vi "Process.vi"(8 "error in":errorcluster, 11 "Inst UI.Attocube-3DR":refnum<class "Inst UI.Attocube-3DR.lvclass">) -> (0 "error out":errorcluster, 3 "Inst UI.Attocube-3DR out":refnum<class "Inst UI.Attocube-3DR.lvclass">)   [LabVIEW 2019, in "Inst UI.Attocube-3DR.lvclass"]
doc: "---------------------------------------------------------------\nJKI State Machine Objects™\nhttp://jki.net/state-machine-objects/\nCopyright (C) 2005-2015, JKI <info@jki.net>\nALL RIGHTS RESERVEDJKI State Machine Objects (SMO) 1.0.0.5\nJKI - JKI\nCopyright (c) 2016, JKI"
uses:
  Inst UI.Attocube-3DR.lvclass
  C:/Program Files (x86)/National Instruments/LabVIEW 2019/vi.lib/JKI/JKI SMO/SMO/SMO.lvclass
  C:/Program Files (x86)/National Instruments/LabVIEW 2019/user.lib/LevyLab/Instrument Framework/SMOs/Instrument UI/Instrument UI.lvclass
  C:/Program Files (x86)/National Instruments/LabVIEW 2019/vi.lib/JKI/JKI SMO/SMO.UI/SMO.UI.lvclass
  Inst.Attocube-3DR/Typedefs/Inst.Attocube-3DR.Inputs--Cluster.ctl
  Inst.Attocube-3DR/Typedefs/Inst.Attocube-3DR.getAll--Cluster.ctl
  Inst.Attocube-3DR/Inst.Attocube-3DR.lvclass
  C:/Program Files (x86)/National Instruments/LabVIEW 2019/user.lib/LevyLab/Instrument Framework/SMOs/Instrument/Instrument.lvclass
  Inst UI.Attocube-3DR.UI--Cluster.ctl
  Inst.Attocube-3DR/Typedefs/Inst.Attocube-3DR.Configuration--Cluster.ctl
  <userlib>/LevyLab/Instrument Framework/SMOs/Configuration/Configuration.lvclass
  <userlib>/LevyLab/Instrument Framework/SMOs/RemoteControl/Typedefs/Message--Cluster.ctl
  <userlib>/LevyLab/Instrument Framework/SMOs/Instrument UI/Instrument UI.lvclass/Instrument UI.ctl
  Inst.Attocube-3DR/Inst.Attocube-3DR.lvclass/Inst.Attocube-3DR.ctl
  <vilib>/JKI/JKI SMO/SMO/SMO.lvclass/SMO.ctl
  <userlib>/LevyLab/Instrument Framework/SMOs/Configuration/Configuration.lvclass/Configuration.ctl
  <userlib>/LevyLab/Instrument Framework/SMOs/Instrument/Instrument.lvclass/Instrument.ctl
  <userlib>/LevyLab/Instrument Framework/SMOs/Instrument/Typedefs/Client Type--Enum.ctl
  862ff513-51e6-4ac6-ad45-748a4df68803.vi
  048e63fc-1edb-448e-8f4f-f5318f48fab1.vi
  6f37eb51-0e53-4202-aa6b-7eeea6d1e979.vi
  436f7c45-6ac9-4282-a393-d7a55f5a58f8.vi
  53aa8742-20c4-45a9-88cf-31145ab324ca.vi
  a7dc0b2d-59f7-45fe-b3a9-fa8b57d3da12.vi
  4acd7b6f-92e7-4c4b-af86-ffc31bbcab9e.vi
  e11c7c74-b7c8-4525-a80a-41ba14629eb8.vi
  b80c2030-d11d-4dfa-959a-d9fba43c27d5.vi
  9f19d11c-c97f-4e63-8b6c-fa81cfd939c9.vi
  a687013f-834b-44a6-a6f3-22fcdf7d7604.vi
  d852ea7b-884f-4206-b538-26d982e90c02.vi
  6e0f0dad-eeb2-4aa9-8821-537bff27e402.vi
  351b4355-bf82-4134-82c7-732762f03f32.vi
  2787704c-df89-403c-943f-ae81abeff9f3.vi
  16be1e38-bb79-47d8-99ba-5a82125cb6c1.vi
  c0fbbb13-e8ef-413d-99ab-b1af3e8c1fc5.vi
  7278661c-b813-447f-a135-8e1ce543f15b.vi
  77de4e95-45da-414c-9291-629979477714.vi
  fc3948ed-5b37-4c89-8f64-66d1f3e9a865.vi
  89faabad-b894-427a-af3b-2e65de9d785f.vi
  6d94cbbf-a9ac-4f89-8b31-e4a871a3db8e.vi
  914930c5-8721-4ac6-bb66-38959b5d5002.vi
  a5ebc035-e685-45b2-a8ec-287c660a7532.vi
  c3992a28-0ace-4d19-8331-9b0e91a8ecb4.vi
  9e101b16-2f91-4f38-b95c-e3ff51136ff6.vi
  99d154c9-cb9c-4973-bc75-571f88aa4a64.vi
  1056dc58-91e4-4912-a0c3-223d5a7ab089.vi
  1b9e2014-56cb-49fc-a14d-f0a40d2771d4.vi
  151c6d9c-9f8f-4aeb-92d7-c211fa7e2556.vi
  b6919943-735e-4033-8b93-0939513f520d.vi
  d99a13ac-48ea-4f37-a989-76a16f5559e3.vi
  f1f28e6d-5397-42c6-984c-224e3dbbef4b.vi
  f68b141c-1cbc-4bee-b372-ea377a2360ca.vi
  32104498-4a8d-4312-9ef2-1fa6833386a6.vi
  f6d8fc86-ed5e-4e4c-a4d2-98ad122425f6.vi
  09e9697b-516c-49fb-b2dc-692589121b6f.vi
  <vilib>/JKI/JKI SMO/SMO/Private/ReftoDVR--SMO.vi
  09e9697b-516c-49fb-b2dc-692589121b6f.vi/3ffc5513-9bd7-4c71-8aef-4de823704d0f.vi
  09e9697b-516c-49fb-b2dc-692589121b6f.vi/3ffc5513-9bd7-4c71-8aef-4de823704d0f.vi/f6b0c238-dc1e-49e3-8a4e-b8369e72da79.vi
  <userlib>/LevyLab/Instrument Framework/SMOs/Instrument/API/Send and Receive.vi
  09e9697b-516c-49fb-b2dc-692589121b6f.vi/3ffc5513-9bd7-4c71-8aef-4de823704d0f.vi/a86054fe-ddd2-4fec-9414-8fc011e039af.vi
  <userlib>/LevyLab/Instrument Framework/SMOs/Instrument/Private/Get Client Type.vi
  09e9697b-516c-49fb-b2dc-692589121b6f.vi/3ffc5513-9bd7-4c71-8aef-4de823704d0f.vi/f6b0c238-dc1e-49e3-8a4e-b8369e72da79.vi/2c6d981d-8b19-4ad3-942a-196c15fa35a5.vi
  09e9697b-516c-49fb-b2dc-692589121b6f.vi/3ffc5513-9bd7-4c71-8aef-4de823704d0f.vi/f6b0c238-dc1e-49e3-8a4e-b8369e72da79.vi/45ea1e73-aa8f-40ed-94ca-4b399240c4c1.vi
  09e9697b-516c-49fb-b2dc-692589121b6f.vi/3ffc5513-9bd7-4c71-8aef-4de823704d0f.vi/a86054fe-ddd2-4fec-9414-8fc011e039af.vi/b596e68e-c0c0-4011-92a4-140a9372dc21.vi
  09e9697b-516c-49fb-b2dc-692589121b6f.vi/3ffc5513-9bd7-4c71-8aef-4de823704d0f.vi/a86054fe-ddd2-4fec-9414-8fc011e039af.vi/f487987f-ebb9-4243-a7de-9c5ef0d70179.vi
  09e9697b-516c-49fb-b2dc-692589121b6f.vi/3ffc5513-9bd7-4c71-8aef-4de823704d0f.vi/a86054fe-ddd2-4fec-9414-8fc011e039af.vi/b596e68e-c0c0-4011-92a4-140a9372dc21.vi/c9a861e6-b5dc-4bd8-be54-56d7304e8390.vi
  09e9697b-516c-49fb-b2dc-692589121b6f.vi/3ffc5513-9bd7-4c71-8aef-4de823704d0f.vi/a86054fe-ddd2-4fec-9414-8fc011e039af.vi/b596e68e-c0c0-4011-92a4-140a9372dc21.vi/402cfb81-c0e6-461e-a8cb-63e9dc5cb757.vi
  <vilib>/JDP Science/JSONtext/Variant to JSON Text.vi
  <userlib>/LevyLab/Instrument Framework/SMOs/Instrument/Private/Get RC Connection Status.vi
  <userlib>/LevyLab/Instrument Framework/SMOs/Instrument/API/Enum to String.vi
  <userlib>/LevyLab/Instrument Framework/SMOs/RemoteControl/API/Send and Receive.vi
  <vilib>/Utility/Data Type/Get Type Information.vi
  <vilib>/JDP Science/JSONtext/JSON text to Variant.vi
  <vilib>/National Instruments/GUID Generator/Guid Generator.vi
  <userlib>/LevyLab/Instrument Framework/SMOs/Instrument/Private/Instrument.MessageFromProcess.EventStructure.vi
  <vilib>/JDP Science/JSONtext/LVClass Serializer/JSONtext LVClass Serializer.lvclass
  <userlib>/LevyLab/Instrument Framework/SMOs/Instrument/Instrument.lvclass
  <userlib>/LevyLab/Instrument Framework/SMOs/Instrument UI/Instrument UI.lvclass
  <vilib>/JKI/JKI SMO/SMO/SMO.lvclass
  <vilib>/JKI/JKI SMO/SMO.UI/SMO.UI.lvclass
  <userlib>/LevyLab/Instrument Framework/SMOs/RemoteControl/RemoteControl.lvclass
  69065371-e868-4e0f-beed-6b6e2b461ff4.vi
  C:/Program Files (x86)/National Instruments/LabVIEW 2019/user.lib/LevyLab/Instrument Framework/Instrument Types/VSource/Instrument.VSource.lvclass
panel:
  in  "Exit":bool
  out "Axis 1: Current Position (°)":i32
  out "Axis 1: rot. count":i32
  out "Axis 1: Capacitance [nF]":i32
  out "Axis 2: Capacitance [nF]":i32
  out "Axis 1: speed (°/s)":i32
  out "Axis 1: StepWidth":i32
  out "Axis 2: StepWidth":i32
  out "Axis 2: speed (°/s)":i32
  out "Axis 2: rot. count":i32
  out "last move time":timestamp
  out "axis 1:\nCurrent position [µm/°/m°] 2":i32(knob) scale=65.0..270.0
  in  "set static amplitude\nwhen moving":bool
  in  "static amplitude (mV)":dbl=2.0 min=0.001 max=2.0 format="%#_13g"
  in  "axis 2:\nStop moving":bool
  in  "axis 1:\nStop moving":bool
  in  "axis 2:\nstop detection":bool
  in  "axis 1:\nstop detection":bool
  in  "axis 2:\nOutput":bool
  in  "axis 1:\ncontrol mode":enum16{"speed", "amplitude", "step size"}(ring)=enum."amplitude"
  in  "axis 2:\ncontrol mode":enum16{"speed", "amplitude", "step size"}(ring)=enum."amplitude"
  in  "axis 1:\nOutput":bool
  in  "axis 2:\ncap. measure":bool
  in  "axis 1:\ncap. measure":bool
  out "axis 2:\nCurrent position [µm/°/m°] 2":i32(knob) scale=5.0..320.0
  in  "axis 2:\nFrequency [Hz]":i32=800 min=0 max=20000 format="%.0fHz"
  in  "axis 1:\nFrequency [Hz]":i32=800 min=0 max=20000 format="%.0fHz"
  in  "axis 2:\nDCLevel [V]":dbl min=0.0 max=140.0 step=0.001 format="%.3f"
  in  "axis 1:\nDCLevel [V]":dbl min=0.0 max=140.0 step=0.001 format="%.3f"
  in  "axis 2:\nAmplitude [V]":dbl=35.0 min=0.0 max=150.0 format="%.3gV"
  in  "axis 1:\nAmplitude [V]":dbl=40.0 min=0.0 max=150.0 format="%.3gV"
  in  "axis 2:\ncontinuous back":bool
  in  "axis 2:\ncontinuous fwd":bool
  in  "axis 1:\ncontinuous back":bool
  in  "axis 1:\ncontinuous fwd":bool
  in  "axis 2:\nsingle step fwd":bool
  in  "axis 2:\nsingle step back":bool
  in  "axis 1:\nsingle step back":bool
  in  "axis 1:\nsingle step fwd":bool
  in  "axis 2:\nsp position °":i32=78 min=5 max=320
  in  "axis 2:\nsp rot count":dbl
  in  "axis 1:\nsp rot count":i32
  in  "axis 1:\nsp position °":dbl=167.0 min=65.0 max=270.0 format="%.4g"
  in  "axis 2:\nAbsolute":bool
  in  "axis 2:\nRelative":bool
  in  "axis 1:\nRelative":bool
  in  "axis 1:\nAbsolute":bool
  in  "axis 1: \nTarget GND":bool
  in  "axis 1:\nSingle Circle Mode":bool
  in  "axis 2:\nSingle Circle Mode":bool
  in  "axis 2: \nTarget GND":bool
  out "axis 2:\npositioner status":T1
  out "axis 2:\nCurrent position (°)":i32
  out "axis 1:\npositioner status":T1
  out "handle":i32=5
  # "Axis 1: large axis"
  # "Axis 2: small axis"
  # "Notes: \n\n***Switch controller to ground (output=false) before connecting the rotator and while cooling down/warming up***\n\nAxis 1 (large axis): Position is limited by physical stops to angles from 65° to 270°\n\nAxis 2 (small axis): Encoded positions are limited to angles from 5° to 320°, not physically limited to one rotation.  Keep single circle mode OFF to limit the rotation count to zero and protect the wiring from over-rotating.\n\nStatic Amplitude: Sets the voltage applied to the resitive readout system.  Range: 0.001 V to 2V.  Higher voltages enhace the sensitivity but lower voltages minimize heat dissipation for low temperature applications.\n\nAbsolute: positioner travels from its current position to      the target position.\n\nTarget Ground: positioner will be grounded when the target position is reached.\n\nSingle circle mode: If OFF absolute and relative positioning are only allowed up to a full circle, keeps rot count at zero.\n\nOutput: When checked, the repective axis output is enabled.  Deactivating sets the axis to GND\n\nControl mode: \n     amplitude: individual steps of the piezo are definied by        the amplitude.  Driven in open-loop mode, travel speed and step width may vary\n     speed: feedback enables a constant travel speed by closed-loop control of the amplitude and frequency.  Speed is set by adjusting the amplitude and/or frequency values.\n     step width: Step size in controlled to a constant value.  Amplitude is closed-loop controlled.  Step width is set by adjusting the amplitude"
  # "Automatic Positioning"
  # "Automatic Positioning"
  # "Manual Positioning"
  # "Manual Positioning"
  # "Move Single Step"
  # "Move Single Step"
  # "Move Continuous"
  # "Move Continuous"
  # "Capacitance Measurement"
  # "Capacitance Measurement"
  # "SMO UI Template"
  # "For instructions on how to use the JKI State Machine Objects, examples and video tutorials, visit:\nhttp://jki.net/state-machine-objects/\n\nJKI State Machine Objects™\nhttp://jki.net/state-machine-objects/\nCopyright (C) 2005-2015, JKI <info@jki.net>\nALL RIGHTS RESERVED"
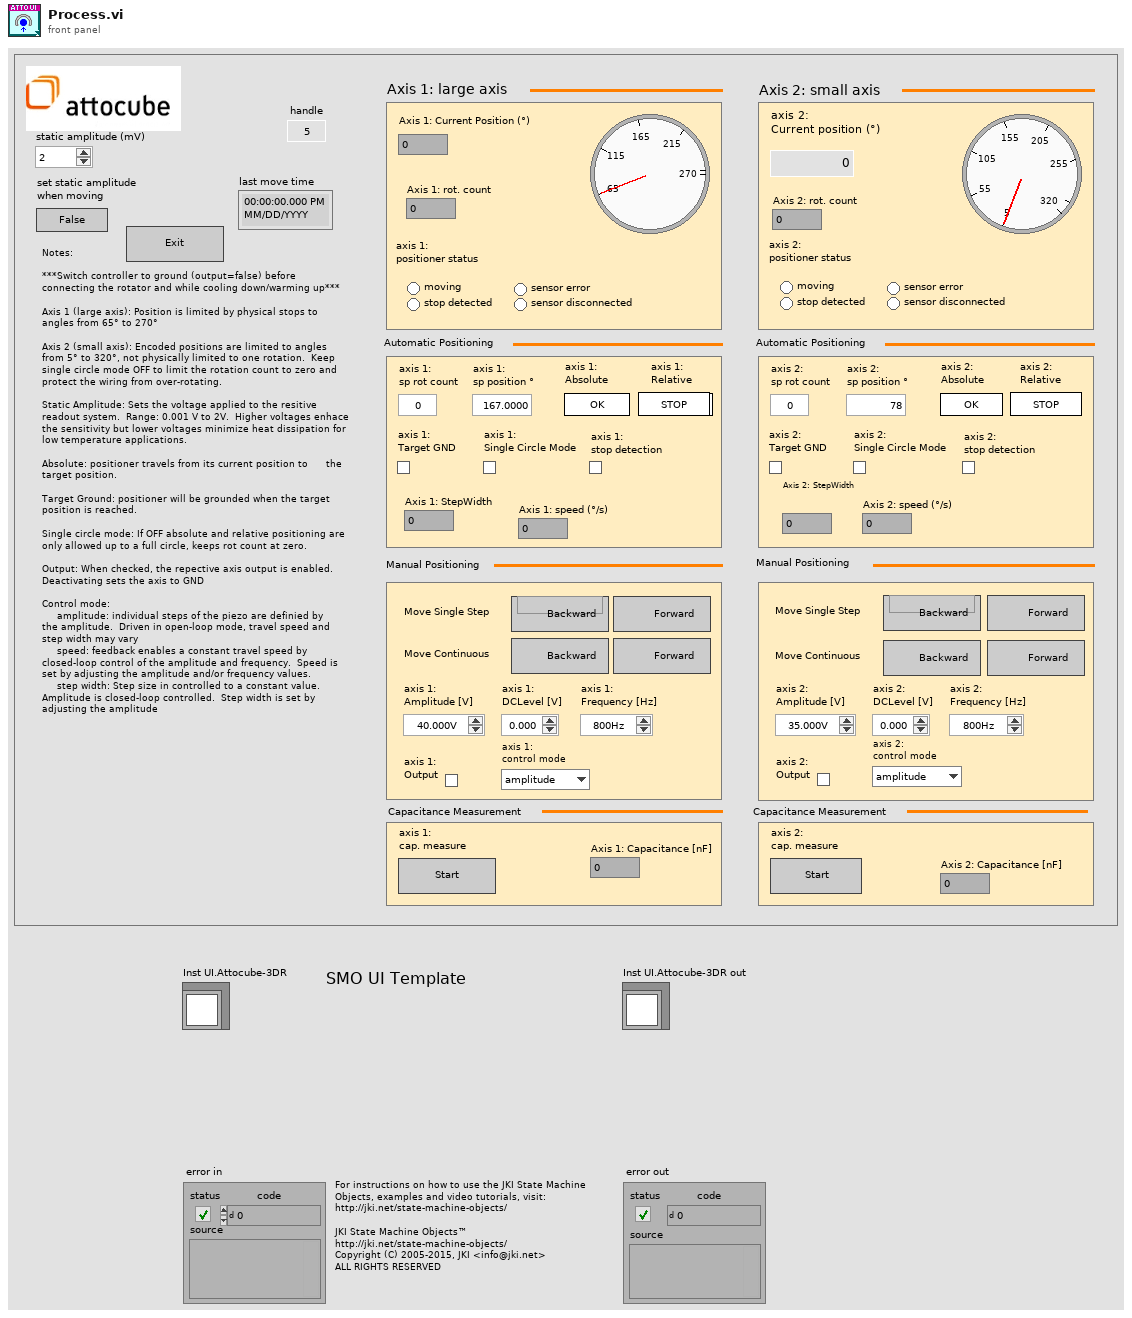
[diagram p1: front panel]
types:
  T1 = cluster{"moving":bool, "stop detected":bool, "sensor error":bool, "sensor disconnected":bool}
  T2 = typedef "Inst.Attocube-3DR.lvclass/Inst.Attocube-3DR.Inputs--Cluster.ctl" = cluster{"Handle":i32, "Axes Number":u8, "Axis 1: sp Position":dbl, "Axis 2: sp Position":dbl, "Axis 1: sp rot count":i32, "Axis 2: sp rot count":i32, "Backward or Forward?":bool, "Axis 1: Amplitude [V] ":dbl, "Axis 2: Amplitude [V] ":dbl, "Axis 1: DCLevel [V]":dbl, "Axis 2: DCLevel [V]":dbl, "Axis 1: Frequency [Hz]":i32, "Axis 2: Frequency [Hz]":i32, "Axis 1:\ncontrol mode":enum16{"speed", "amplitude", "step size"}, "Axis 2:\ncontrol mode":enum16{"speed", "amplitude", "step size"}, "axis 1:\nOutput":bool, "axis 2:\nOutput 2":bool, "axis 1:\nstop detection":bool, "axis 2:\nstop detection":bool, "axis 1:\nSingle Circle Mode":bool, "axis 2:\nSingle Circle Mode":bool, "axis 1: \nTarget GND":bool, "axis 2: \nTarget GND":bool, "Set static Amplitude when moving?":bool, "Static Amplitude (mV)":dbl}
  T3 = enum32{"invalid app kind", "Development System", "Run Time System", "Student Edition", "Embedded LabVIEW", "Evaluation", "Custom"}
  T4 = enum32{"Invalid", "Standard", "Closed", "Hidden", "Minimized", "Maximized"}
  T5 = typedef "Instrument.lvclass/Client Type--Enum.ctl" = enum16{"Remote", "Local"}
  T6 = typedef "Inst.Attocube-3DR.lvclass/Inst.Attocube-3DR.Configuration--Cluster.ctl" = cluster{"Example Setting 1":dbl, "Example Setting 2":dbl, "Example Setting 3":string}
  T7 = typedef "Inst.Attocube-3DR.lvclass/Inst.Attocube-3DR.getAll--Cluster.ctl" = cluster{"Axis 1: Amplitude":i32, "Axis 1: Capacitance":i32, "Axis 1: Current Position":i32, "Axis 1: DCLevel":i32, "Axis 1: Frequency":i32, "Axis 1: StepWidth":i32, "Axis 1: control mode":i32, "Axis 1: rot. count":i32, "Axis 1: sp position":i32, "Axis 1: sp rot. count":i32, "Axis 1: speed":i32, "Axis 1: Target GND":bool, "Axis 1: Output":bool, "Axis 1: Single Circle Mode":bool, "Axis 1: moving":bool, "Axis 1: stop detected":bool, "Axis 1:  sensor error":bool, "Axis 1: sensor diconnected":bool, "Axis 1: stop enable":bool, "Axis 2: Current Position":i32, "Axis 2: DCLevel":i32, "Axis 2: Frequency":i32, "Axis 2: StepWidth":i32, "Axis 2: control mode":i32, "Axis 2: rot. count":i32, "Axis 2: sp position":i32, "Axis 2: sp rot. count":i32, "Axis 2: speed":i32, "Axis 2: Capacitance":i32, "Axis 2: Amplitude":i32, "Axis 2: Target GND":bool, "Axis 2: Output":bool, "Axis 2: Single Circle Mode":bool, "Axis 2: moving":bool, "Axis 2: stop detected":bool, "Axis 2:  sensor error":bool, "Axis 2: sensor diconnected":bool, "Axis 2: stop enable":bool}
  T8 = typedef "Inst UI.Attocube-3DR.lvclass/Inst UI.Attocube-3DR.UI--Cluster.ctl" = cluster{"static amplitude (mV)":dbl, "Axis1":cluster{"axis 1:\nsp rot count":i32, "axis 1:\nsp position °":dbl, "axis 1:\nAmplitude [V]":dbl, "axis 1:\nDCLevel [V]":dbl, "axis 1:\nFrequency [Hz]":i32}, "Axis2":cluster{"axis 2:\nsp rot count":i32, "axis2:\nsp position °":dbl, "axis 2:\nAmplitude [V]":dbl, "axis 2:\nDCLevel [V]":dbl, "axis 2:\nFrequency [Hz]":i32}}
  T9 = typedef "RemoteControl.lvclass/Message--Cluster.ctl" = cluster{"Command":string, "Data":variant, "ID":string}
  T10 = cluster{"Core":cluster{"Current VI Reference":refnum<vi>, "Close Panel on Exit?":bool, "Last Error":cluster{"error":errorcluster, "previous state":string, "remaining states":string}, "Shutdown?":bool}, "Instrument UI":refnum<class "Inst UI.Attocube-3DR.lvclass">, "Instrument":refnum<class "Inst.Attocube-3DR.lvclass">, "Configuration":refnum<class "Configuration.lvclass">, "Config Cluster":T6, "getAll":T7, "UI Cluster":T8, "Message":T9}
  T11 = cluster{"Current VI Reference":refnum<vi>, "Close Panel on Exit?":bool, "Last Error":cluster{"error":errorcluster, "previous state":string, "remaining states":string}, "Shutdown?":bool}
  T12 = cluster{"Axis 1: moving":bool, "Axis 1: stop detected":bool, "Axis 1:  sensor error":bool, "Axis 1: sensor diconnected":bool}
  T13 = cluster{"Axis 2: moving":bool, "Axis 2: stop detected":bool, "Axis 2:  sensor error":bool, "Axis 2: sensor diconnected":bool}
  T14 = typedef "SMO.lvclass/Protected Events.ctl" = cluster{"StopProcesses":refnum<user-event>, "AbortProcesses":refnum<user-event>, "Config Changed":refnum<user-event>, "Dependency":refnum<user-event>}
  T15 = typedef "Instrument.lvclass/PublicEvents--Cluster.ctl" = cluster{"MessageFromProcess":refnum<user-event>}
  T16 = typedef "Inst.Attocube-3DR.lvclass/PublicEvents--Cluster.ctl" = cluster{"MessageFromProcess":refnum<user-event>}
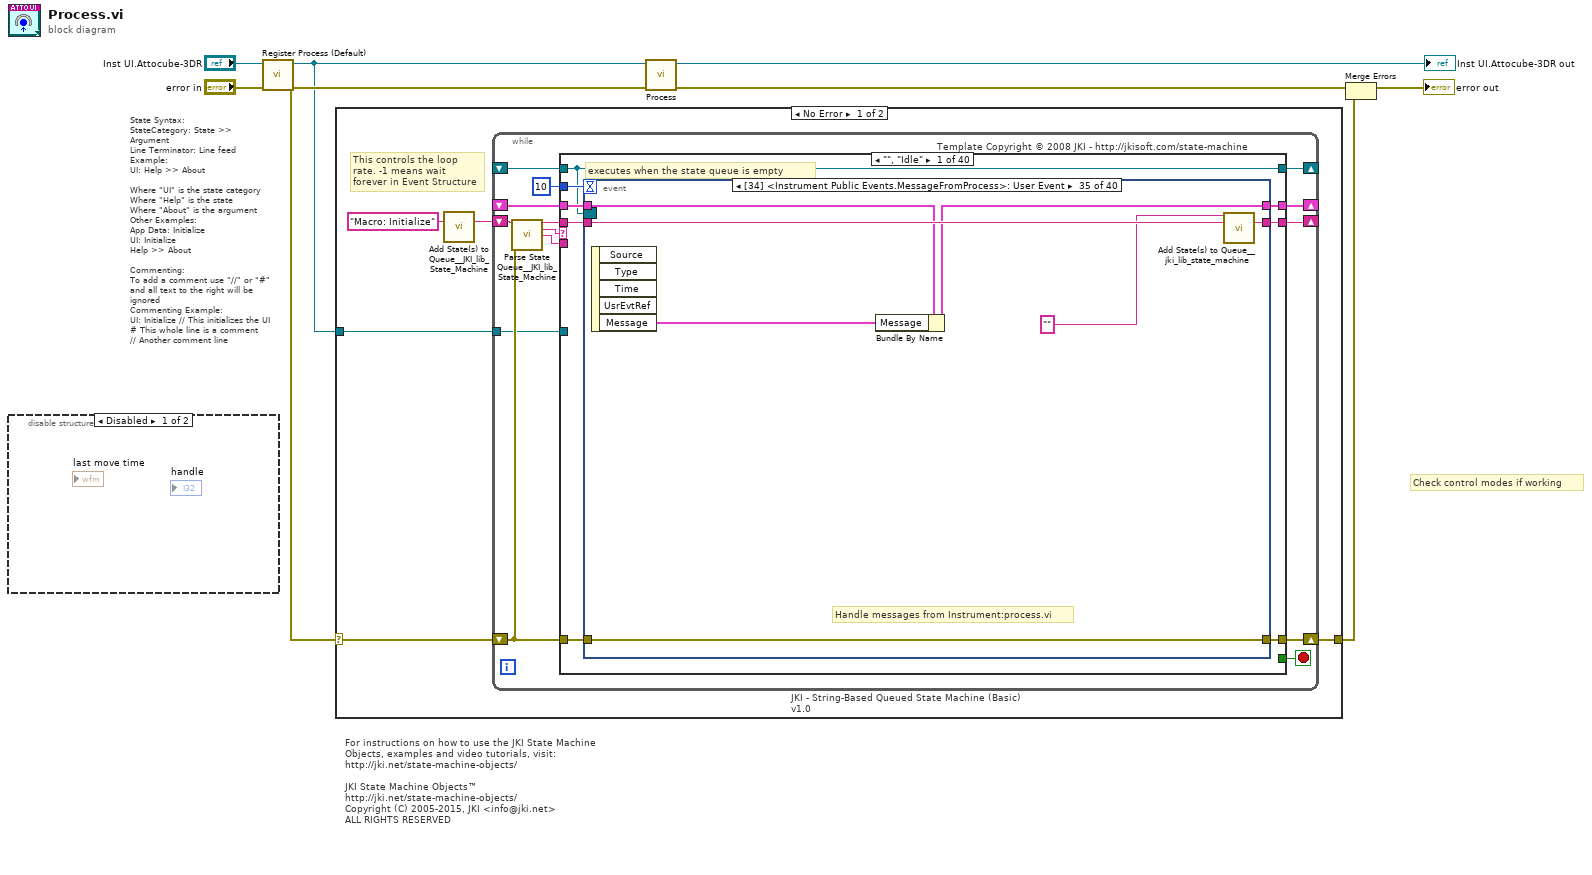
[diagram p0: block diagram]
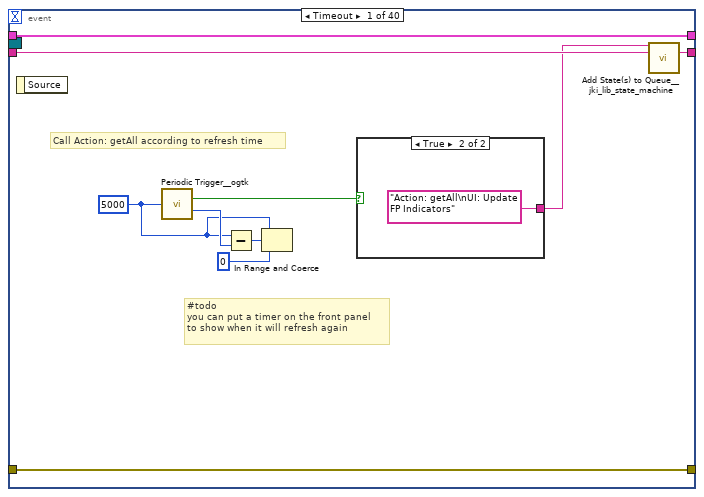
[diagram p3: hidden frame]
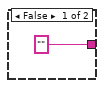
[diagram p4: hidden frame]
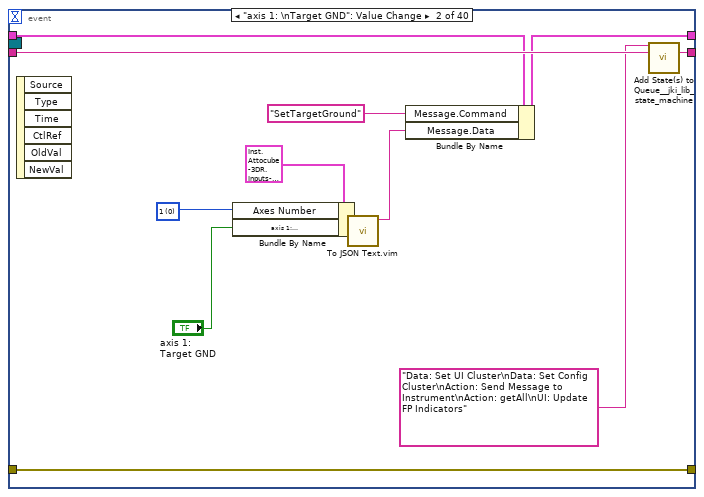
[diagram p5: hidden frame]
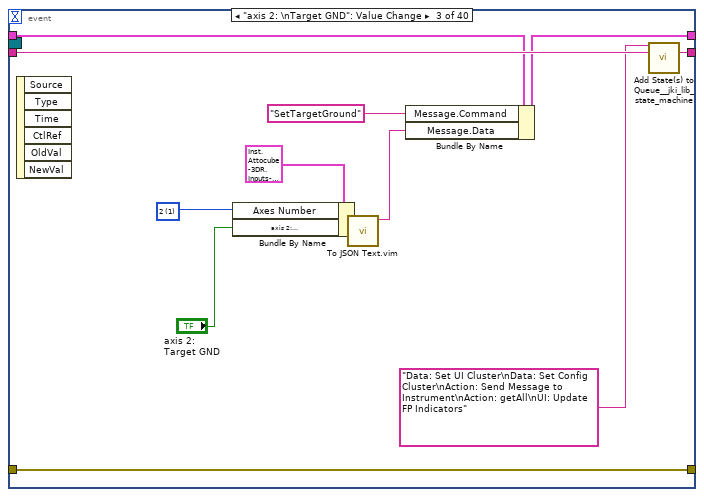
[diagram p6: hidden frame]
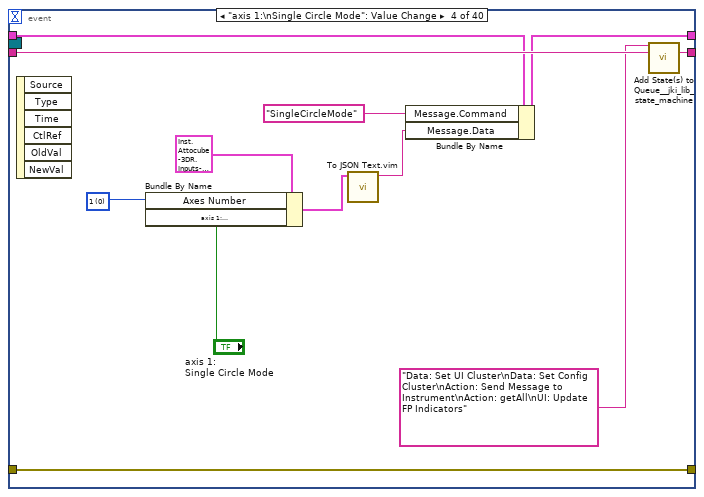
[diagram p7: hidden frame]
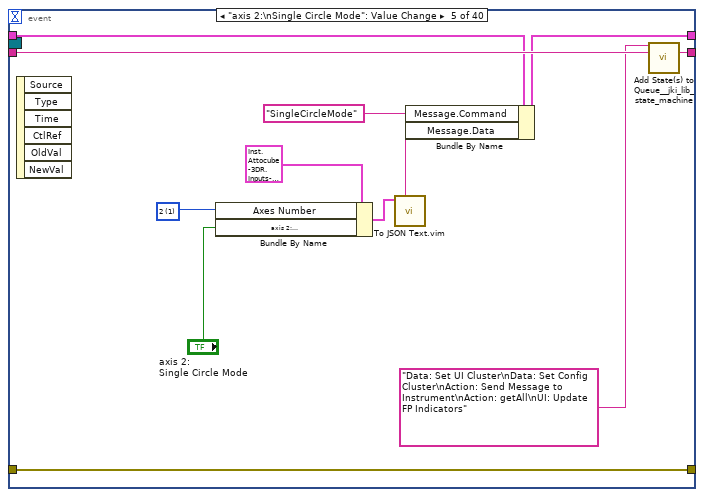
[diagram p8: hidden frame]
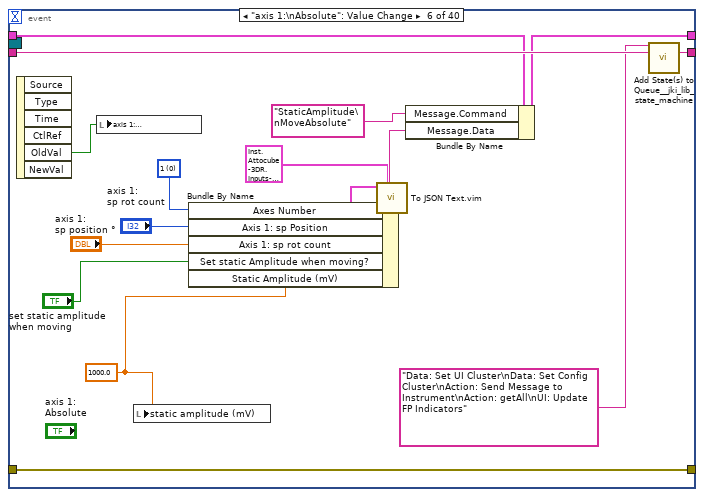
[diagram p9: hidden frame]
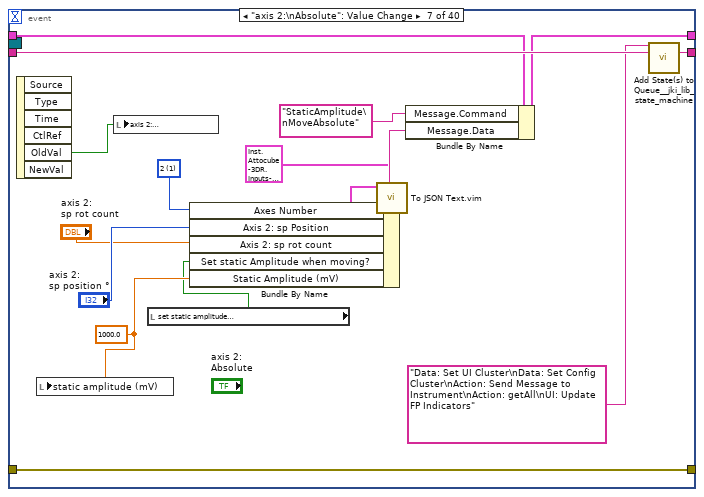
[diagram p10: hidden frame]
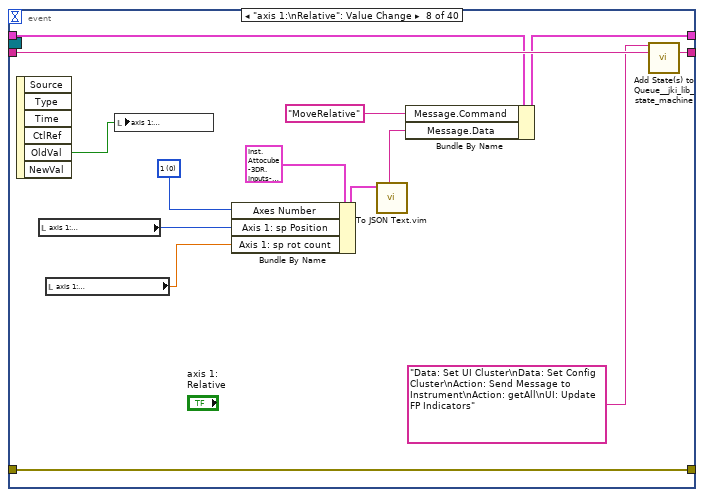
[diagram p11: hidden frame]
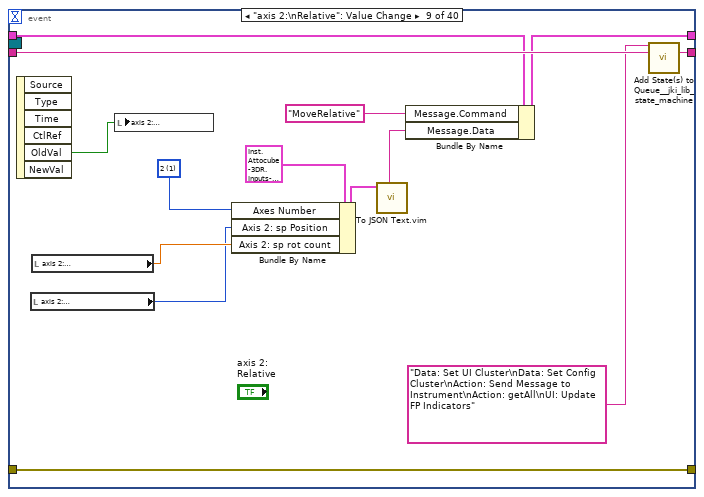
[diagram p12: hidden frame]
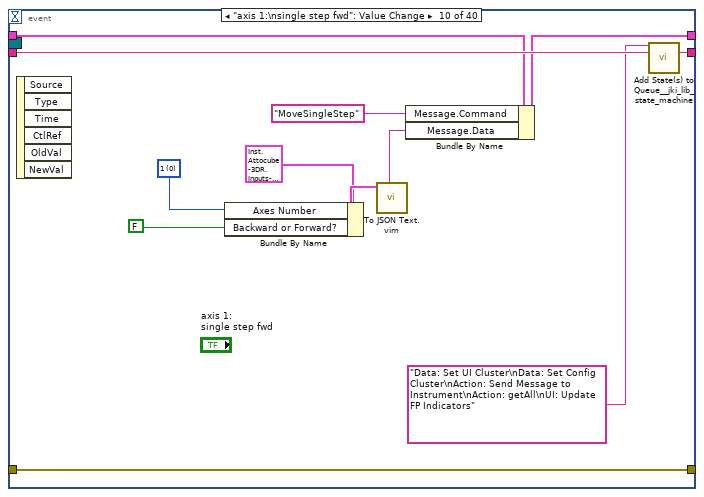
[diagram p13: hidden frame]
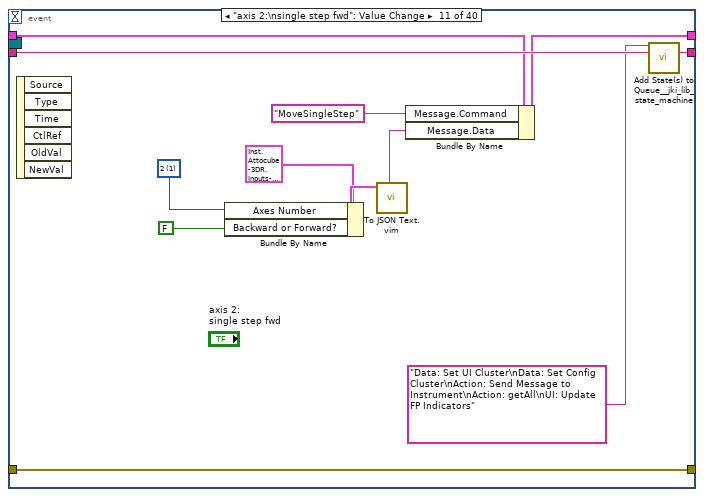
[diagram p14: hidden frame]
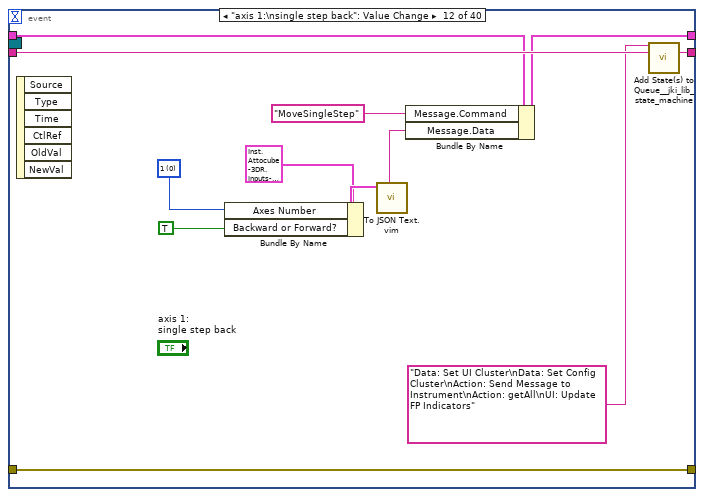
[diagram p15: hidden frame]
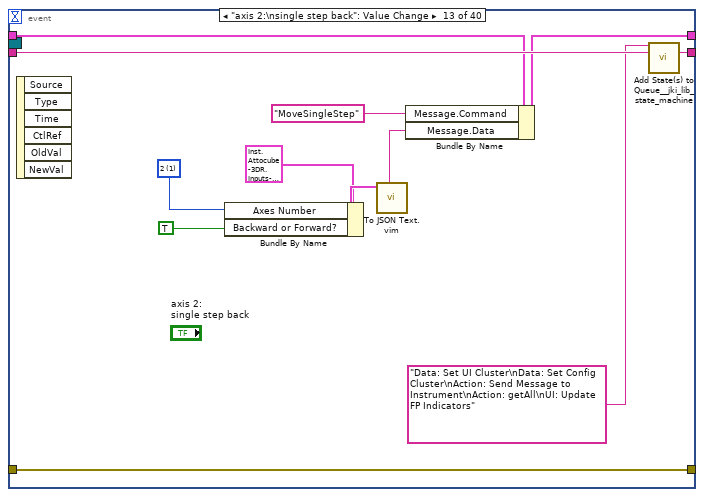
[diagram p16: hidden frame]
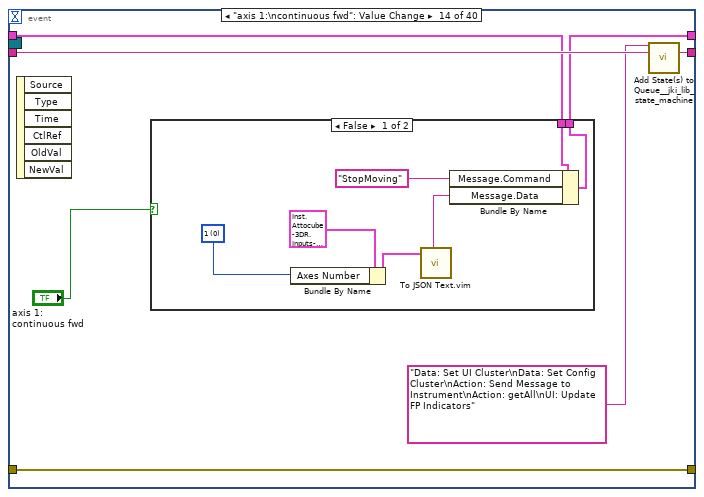
[diagram p17: hidden frame]
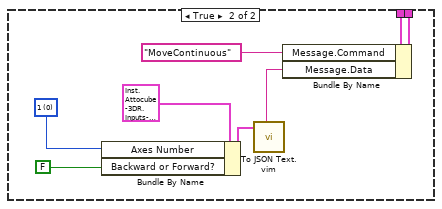
[diagram p18: hidden frame]
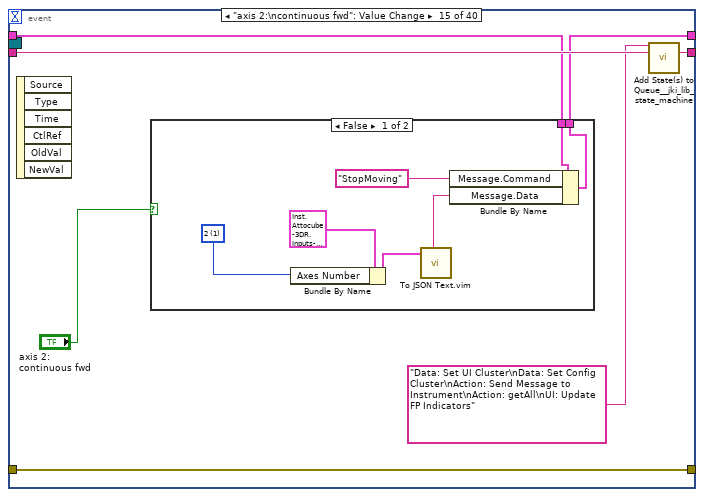
[diagram p19: hidden frame]
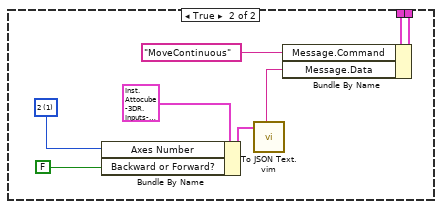
[diagram p20: hidden frame]
diagram:
  # "Check control modes if working"
  # "State Syntax:\nStateCategory: State >> Argument\nLine Terminator: Line feed\nExample:\nUI: Help >> About\n\nWhere \"UI\" is the state category\nWhere \"Help\" is the state\nWhere \"About\" is the argument\nOther Examples:\nApp Data: Initialize\nUI: Initialize\nHelp >> About\n\nCommenting:\nTo add a comment use \"//\" or \"#\" and all text to the right will be ignored\nCommenting Example:\nUI: Initialize // This initializes the UI\n# This whole line is a comment\n// Another comment line"
  # "For instructions on how to use the JKI State Machine Objects, examples and video tutorials, visit:\nhttp://jki.net/state-machine-objects/\n\nJKI State Machine Objects™\nhttp://jki.net/state-machine-objects/\nCopyright (C) 2005-2015, JKI <info@jki.net>\nALL RIGHTS RESERVED"
  n1 = disable-structure shown="Disabled" {
    frame Disabled {
    }
    frame Enabled {
    }
  }
  n2 = call <vilib>:"Register Process (Default).vi"("error in (no error)"="error in", "SMO"="Inst UI.Attocube-3DR") -> ("error out"=w5:errorcluster, "SelfRef"=w4:refnum<class "Inst UI.Attocube-3DR.lvclass">)  [unwired: 8 in]
  n3 = case shown="No Error" w5 {
    selector: w5 -> [w10 w967]
    tunnel: w4 -> [w11 _]
    tunnel: [w9 w967] -> w1
    frame No Error {
      # "This controls the loop rate. -1 means wait forever in Event Structure"
      n4 = call <vilib>:"Add State(s) to Queue__JKI_lib_State_Machine.vi"("State(s) in (\"\")"="Macro: Initialize") -> ("States Out"=w13:string)  [unwired: 14 in]
      n5 = while "JKI - String-Based Queued State Machine (Basic) v1.0" {
        shift-right: [w20] -> _
        shift-left: _ -> [w19]
        shift-right: [w23] -> w9
        shift-left: w10 -> [w17]
        shift-right: [w22] -> _
        shift-left: w13 -> [w24]
        tunnel: w11 -> [w16]
        shift-right: [w15] -> _
        shift-left: _ -> [w14]
        stop <- w21 stop-if-true
        # "Template Copyright © 2008 JKI - http://jkisoft.com/state-machine"
        n6 = call <vilib>:"Parse State Queue__JKI_lib_State_Machine.vi"("State Queue"=w24, "Error In (no error)"=w17) -> ("Remaining States"=w26:string, "Current State"=w27:string, "Arguments"=w25:string)  [unwired: 11 in]
        n7 = case shown="\"\", \"Idle\"" w27 {
          selector: w27 -> [_ _ w537 _ _ _ _ _ _ _ _ _ _ _ _ _ _ _ _ _ _ _ _ _ _ _ _ _ _ _ _ _ _ _ _ _ _ _ _ _]
          tunnel: w26 -> [w35 w535 w541 w560 w564 w579 w584 w602 w619 w627 w634 w639 w646 w662 w696 w703 w719 w751 w760 w772 w782 w788 w803 w808 w819 w826 w831 w847 w853 w858 w873 w881 w893 w900 w907 w919 w932 w942 w954 w966]
          tunnel: w25 -> [_ _ _ _ _ _ _ _ _ _ _ _ _ _ _ w697 w713 _ _ _ _ _ _ _ _ _ _ _ _ _ _ _ _ _ _ _ _ _ _ _]
          tunnel: w19 -> [w33 w532 w539 w551 w567 w575 w581 _ w613 w623 w628 w636 w644 w655 w691 w701 w715 w748 w756 w762 w779 w785 w790 w805 w816 w821 w828 w845 w851 w855 w866 w878 w884 w895 w901 w911 w926 w934 w949 w961]
          tunnel: [w32 w533 w543 w557 w569 w574 w582 w589 w617 w625 w630 w637 w641 w660 w692 w698 w716 w749 w758 w770 w780 w786 w801 w806 w810 w822 w829 w842 w848 w856 w859 w876 w885 w897 w902 w916 w929 w939 w945 w957] -> w23
          tunnel: w17 -> [w31 w533 w542 w557 w563 _ w582 w586 w617 w625 w631 w637 w642 w660 w692 w699 w717 w749 w758 w770 w780 w786 w801 w806 w811 w823 w829 w832 w849 w856 w868 w874 w886 w897 w903 w912 w921 w935 w946 w958]
          tunnel: [w34 w534 w540 w559 w561 w578 w583 w601 w618 w626 w633 w638 w645 w661 w695 w702 w718 w750 w759 w771 w781 w787 w802 w807 w818 w825 w830 w846 w852 w857 w872 w880 w892 w899 w906 w918 w931 w941 w953 w965] -> w22
          tunnel: [_ _ _ _ _ TRUE _ _ _ _ _ _ _ _ _ _ _ _ _ _ _ _ _ _ _ _ _ _ _ _ _ _ _ _ _ _ _ _ _ _] -> w21
          tunnel: [w30 w532 w539 w558 w566 w575 w581 w600 w615 w622 w628 w636 w644 w655 w691 w701 w715 w748 w756 w763 w779 w785 w790 w805 w816 w821 w828 w845 w851 w855 w870 w878 w882 w894 w901 w913 w927 w936 w950 w962] -> w20
          tunnel: 10 ("Timeout") -> [w29 _ _ _ _ _ _ _ _ _ _ _ _ _ _ _ _ _ _ _ _ _ _ _ _ _ _ _ _ _ _ _ _ _ _ _ _ _ _ _]
          tunnel: w16 -> [_ _ _ _ _ _ _ w587 _ _ _ _ _ _ _ _ _ _ _ _ _ _ _ _ _ _ _ _ _ _ _ _ _ _ _ _ _ _ _ _]
          tunnel: [w28 w531 w536 w548 w573 w576 w580 w599 w616 w624 w629 w635 w643 w659 w694 w700 w712 w747 w757 w769 w778 w784 w795 w804 w817 w824 w827 w844 w850 w854 w871 w879 w891 w898 w905 w917 w930 w940 w952 w964] -> w15
          tunnel: w14 -> [w28 w531 w536 w548 w573 w576 w580 w599 w616 w624 w629 w635 w643 w659 w694 w700 w712 w747 w757 w769 w778 w784 w795 w804 w817 w824 w827 _ w850 w854 w871 w879 w891 w898 w905 w917 w930 w940 w952 w964]
          frame "", "Idle" {
            # "executes when the state queue is empty"
            n8 = event shown="[34] <Instrument Public Events.MessageFromProcess>: User Event" {
              selector: w28 -> [_ _ _ _ _ _ _ _ _ _ _ _ _ _ _ _ _ _ _ _ _ _ _ _ _ _ _ _ _ _ _ _ _ _ _ _ _ _ _ _]
              dyn-events: _ -> [_ _ _ _ _ _ _ _ _ _ _ _ _ _ _ _ _ _ _ _ _ _ _ _ _ _ _ _ _ _ _ _ _ _ _ _ _ _ _ _]
              timeout: w29 -> [_ _ _ _ _ _ _ _ _ _ _ _ _ _ _ _ _ _ _ _ _ _ _ _ _ _ _ _ _ _ _ _ _ _ _ _ _ _ _ _]
              tunnel: w35 -> [w45 w59 w71 w83 w95 w111 w127 w141 w155 w167 w179 w191 w203 w210 w232 w254 w276 w303 w315 w327 w339 w351 w363 w374 w385 w397 w409 w421 w433 w445 w457 w468 w479 w491 w498 w505 w511 w516 w521 w530]
              tunnel: [w44 w58 w70 w82 w94 w110 w126 w140 w154 w166 w178 w190 w202 w209 w231 w253 w275 w302 w314 w326 w338 w350 w362 w373 w384 w396 w408 w420 w432 w444 w456 w467 w478 w490 w497 w504 w510 w515 w520 w529] -> w34
              tunnel: w33 -> [w42 w51 w63 w76 w87 w103 w119 w133 w147 w159 w171 w183 w195 w205 w227 w249 w271 w295 w307 w319 w331 w343 w355 w366 w377 w389 w401 w413 w425 w437 w449 w460 w471 w483 w495 w502 w507 w513 w518 w527]
              tunnel: [w43 w57 w69 w81 w93 w109 w125 w139 w153 w165 w177 w189 w201 w208 w230 w252 w274 w301 w313 w325 w337 w349 w361 w372 w383 w395 w407 w419 w431 w443 w455 w466 w477 w489 w496 w503 w506 w514 w519 w528] -> w32
              tunnel: w31 -> [w43 w57 w69 w81 w93 w109 w125 w139 w153 w165 w177 w189 w201 w208 w230 w252 w274 w301 w313 w325 w337 w349 w361 w372 w383 w395 w407 w419 w431 w443 w455 w466 w477 w489 w496 w503 w506 w514 w519 w528]
              tunnel: [w42 w52 w64 w77 w88 w104 w120 w134 w148 w160 w172 w184 w196 w206 w228 w250 w272 w296 w308 w320 w332 w344 w356 w367 w378 w390 w402 w414 w426 w438 w450 w461 w472 w484 w494 w501 w507 w513 w518 w527] -> w30
              event Timeout {
                w37 = u32 5000 ("time (ms)")
                # "#todo\nyou can put a timer on the front panel\nto show when it will refresh again"
                # "Call Action: getAll according to refresh time"
                n9 = event-data() -> ()  [unwired: 1 in, 1 out]
                n10 = call <userlib>:"Periodic Trigger__ogtk.vi"("time (ms)"=w37) -> ("Triggered"=w40:bool, "timer value"=w39:u32)  [unwired: 12 in, 1 out]
                n11 = Subtract(x=w37, y=w39) -> (x-y=w38:u32)
                n12 = In Range and Coerce(upper limit=w37, x=w38, lower limit=u32 0) -> ()  [unwired: 2 out]
                n13 = case shown="True" w40 {
                  tunnel: ["" ("State(s) in Front (\"\")") "Action: getAll\nUI: Update FP Indicators" ("State(s) in Front (\"\")")] -> w41
                  frame False {
                  }
                  frame True {
                  }
                }
                n14 = call <vilib>:"Add State(s) to Queue__jki_lib_state_machine.vi"("State(s) in Front (\"\")"=w41, "State(s) in (\"\")"=w45) -> ("States Out"=w44:string)  [unwired: 13 in]
              }
              event "axis 1: \nTarget GND": Value Change {
                w49 = u8 0 items=["1", "2", "3", "4", "5", "6", "7", "8", "9"] ("axis no")
                n15 = event-data() -> ()  [unwired: 1 in, 6 out]
                n16 = Bundle By Name(cluster=T2 {"Handle"=0, "Axes Number"=0, "Axis 1: sp Position"=0.0, "Axis 2: sp Position"=0.0, "Axis 1: sp rot count"=0, "Axis 2: sp rot count"=0, "Backward or Forward?"=FALSE, "Axis 1: Amplitude [V] "=0.0, "Axis 2: Amplitude [V] "=0.0, "Axis 1: DCLevel [V]"=0.0, "Axis 2: DCLevel [V]"=0.0, "Axis 1: Frequency [Hz]"=0, "Axis 2: Frequency [Hz]"=0, "Axis 1:\ncontrol mode"=enum."amplitude", "Axis 2:\ncontrol mode"=enum."amplitude", "axis 1:\nOutput"=FALSE, "axis 2:\nOutput 2"=FALSE, "axis 1:\nstop detection"=FALSE, "axis 2:\nstop detection"=FALSE, "axis 1:\nSingle Circle Mode"=FALSE, "axis 2:\nSingle Circle Mode"=FALSE, "axis 1: \nTarget GND"=FALSE, "axis 2: \nTarget GND"=FALSE, "Set static Amplitude when moving?"=FALSE, "Static Amplitude (mV)"=0.0} ("Inputs"), "Axes Number"=w49, "axis 1: \nTarget GND"="axis 1: \nTarget GND") -> (w54:T2)
                n17 = call "To JSON Text.vim"("Anything"=w54) -> ("<JSON>"=w53:string)  [unwired: 9 in, 1 out]
                n18 = Bundle By Name(cluster=w51, "Message.Command"="SetTargetGround", "Message.Data"=w53) -> (w52:T10)
                n19 = call <vilib>:"Add State(s) to Queue__jki_lib_state_machine.vi"("State(s) in Front (\"\")"="Data: Set UI Cluster\nData: Set Config Cluster\nAction: Send Message to Instrument\nAction: getAll\nUI: Update FP Indicators" ("State(s) in Front (\"\")"), "State(s) in (\"\")"=w59) -> ("States Out"=w58:string)  [unwired: 13 in]
              }
              event "axis 2: \nTarget GND": Value Change {
                w61 = u8 1 items=["1", "2", "3", "4", "5", "6", "7", "8", "9"] ("axis no")
                n20 = event-data() -> ()  [unwired: 1 in, 6 out]
                n21 = Bundle By Name(cluster=T2 {"Handle"=0, "Axes Number"=0, "Axis 1: sp Position"=0.0, "Axis 2: sp Position"=0.0, "Axis 1: sp rot count"=0, "Axis 2: sp rot count"=0, "Backward or Forward?"=FALSE, "Axis 1: Amplitude [V] "=0.0, "Axis 2: Amplitude [V] "=0.0, "Axis 1: DCLevel [V]"=0.0, "Axis 2: DCLevel [V]"=0.0, "Axis 1: Frequency [Hz]"=0, "Axis 2: Frequency [Hz]"=0, "Axis 1:\ncontrol mode"=enum."amplitude", "Axis 2:\ncontrol mode"=enum."amplitude", "axis 1:\nOutput"=FALSE, "axis 2:\nOutput 2"=FALSE, "axis 1:\nstop detection"=FALSE, "axis 2:\nstop detection"=FALSE, "axis 1:\nSingle Circle Mode"=FALSE, "axis 2:\nSingle Circle Mode"=FALSE, "axis 1: \nTarget GND"=FALSE, "axis 2: \nTarget GND"=FALSE, "Set static Amplitude when moving?"=FALSE, "Static Amplitude (mV)"=0.0} ("Inputs"), "Axes Number"=w61, "axis 2: \nTarget GND"="axis 2: \nTarget GND") -> (w66:T2)
                n22 = call "To JSON Text.vim"("Anything"=w66) -> ("<JSON>"=w65:string)  [unwired: 9 in, 1 out]
                n23 = Bundle By Name(cluster=w63, "Message.Command"="SetTargetGround", "Message.Data"=w65) -> (w64:T10)
                n24 = call <vilib>:"Add State(s) to Queue__jki_lib_state_machine.vi"("State(s) in Front (\"\")"="Data: Set UI Cluster\nData: Set Config Cluster\nAction: Send Message to Instrument\nAction: getAll\nUI: Update FP Indicators" ("State(s) in Front (\"\")"), "State(s) in (\"\")"=w71) -> ("States Out"=w70:string)  [unwired: 13 in]
              }
              event "axis 1:\nSingle Circle Mode": Value Change {
                w74 = u8 0 items=["1", "2", "3", "4", "5", "6", "7", "8", "9"] ("axis no")
                n25 = event-data() -> ()  [unwired: 1 in, 6 out]
                n26 = Bundle By Name(cluster=T2 {"Handle"=0, "Axes Number"=0, "Axis 1: sp Position"=0.0, "Axis 2: sp Position"=0.0, "Axis 1: sp rot count"=0, "Axis 2: sp rot count"=0, "Backward or Forward?"=FALSE, "Axis 1: Amplitude [V] "=0.0, "Axis 2: Amplitude [V] "=0.0, "Axis 1: DCLevel [V]"=0.0, "Axis 2: DCLevel [V]"=0.0, "Axis 1: Frequency [Hz]"=0, "Axis 2: Frequency [Hz]"=0, "Axis 1:\ncontrol mode"=enum."amplitude", "Axis 2:\ncontrol mode"=enum."amplitude", "axis 1:\nOutput"=FALSE, "axis 2:\nOutput 2"=FALSE, "axis 1:\nstop detection"=FALSE, "axis 2:\nstop detection"=FALSE, "axis 1:\nSingle Circle Mode"=FALSE, "axis 2:\nSingle Circle Mode"=FALSE, "axis 1: \nTarget GND"=FALSE, "axis 2: \nTarget GND"=FALSE, "Set static Amplitude when moving?"=FALSE, "Static Amplitude (mV)"=0.0} ("Inputs"), "Axes Number"=w74, "axis 1:\nSingle Circle Mode"="axis 1:\nSingle Circle Mode") -> (w72:T2)
                n27 = call "To JSON Text.vim"("Anything"=w72) -> ("<JSON>"=w78:string)  [unwired: 9 in, 1 out]
                n28 = Bundle By Name(cluster=w76, "Message.Command"="SingleCircleMode", "Message.Data"=w78) -> (w77:T10)
                n29 = call <vilib>:"Add State(s) to Queue__jki_lib_state_machine.vi"("State(s) in Front (\"\")"="Data: Set UI Cluster\nData: Set Config Cluster\nAction: Send Message to Instrument\nAction: getAll\nUI: Update FP Indicators" ("State(s) in Front (\"\")"), "State(s) in (\"\")"=w83) -> ("States Out"=w82:string)  [unwired: 13 in]
              }
              event "axis 2:\nSingle Circle Mode": Value Change {
                w85 = u8 1 items=["1", "2", "3", "4", "5", "6", "7", "8", "9"] ("axis no")
                n30 = event-data() -> ()  [unwired: 1 in, 6 out]
                n31 = Bundle By Name(cluster=T2 {"Handle"=0, "Axes Number"=0, "Axis 1: sp Position"=0.0, "Axis 2: sp Position"=0.0, "Axis 1: sp rot count"=0, "Axis 2: sp rot count"=0, "Backward or Forward?"=FALSE, "Axis 1: Amplitude [V] "=0.0, "Axis 2: Amplitude [V] "=0.0, "Axis 1: DCLevel [V]"=0.0, "Axis 2: DCLevel [V]"=0.0, "Axis 1: Frequency [Hz]"=0, "Axis 2: Frequency [Hz]"=0, "Axis 1:\ncontrol mode"=enum."amplitude", "Axis 2:\ncontrol mode"=enum."amplitude", "axis 1:\nOutput"=FALSE, "axis 2:\nOutput 2"=FALSE, "axis 1:\nstop detection"=FALSE, "axis 2:\nstop detection"=FALSE, "axis 1:\nSingle Circle Mode"=FALSE, "axis 2:\nSingle Circle Mode"=FALSE, "axis 1: \nTarget GND"=FALSE, "axis 2: \nTarget GND"=FALSE, "Set static Amplitude when moving?"=FALSE, "Static Amplitude (mV)"=0.0} ("Inputs"), "Axes Number"=w85, "axis 2:\nSingle Circle Mode"="axis 2:\nSingle Circle Mode") -> (w90:T2)
                n32 = call "To JSON Text.vim"("Anything"=w90) -> ("<JSON>"=w89:string)  [unwired: 9 in, 1 out]
                n33 = Bundle By Name(cluster=w87, "Message.Command"="SingleCircleMode", "Message.Data"=w89) -> (w88:T10)
                n34 = call <vilib>:"Add State(s) to Queue__jki_lib_state_machine.vi"("State(s) in Front (\"\")"="Data: Set UI Cluster\nData: Set Config Cluster\nAction: Send Message to Instrument\nAction: getAll\nUI: Update FP Indicators" ("State(s) in Front (\"\")"), "State(s) in (\"\")"=w95) -> ("States Out"=w94:string)  [unwired: 13 in]
              }
              event "axis 1:\nAbsolute": Value Change {
                w97 = 1000.0 ("static amplitude (mV)")
                w101 = u8 0 items=["1", "2", "3", "4", "5", "6", "7", "8", "9"] ("axis no")
                n35 = event-data() -> ("OldVal"=w98:bool)  [unwired: 1 in, 5 out]
                n36 = local write "axis 1:\nAbsolute"(w98) -> ()
                n37 = local write "static amplitude (mV)"(w97) -> ()
                n38 = Bundle By Name(cluster=T2 {"Handle"=0, "Axes Number"=0, "Axis 1: sp Position"=0.0, "Axis 2: sp Position"=0.0, "Axis 1: sp rot count"=0, "Axis 2: sp rot count"=0, "Backward or Forward?"=FALSE, "Axis 1: Amplitude [V] "=0.0, "Axis 2: Amplitude [V] "=0.0, "Axis 1: DCLevel [V]"=0.0, "Axis 2: DCLevel [V]"=0.0, "Axis 1: Frequency [Hz]"=0, "Axis 2: Frequency [Hz]"=0, "Axis 1:\ncontrol mode"=enum."amplitude", "Axis 2:\ncontrol mode"=enum."amplitude", "axis 1:\nOutput"=FALSE, "axis 2:\nOutput 2"=FALSE, "axis 1:\nstop detection"=FALSE, "axis 2:\nstop detection"=FALSE, "axis 1:\nSingle Circle Mode"=FALSE, "axis 2:\nSingle Circle Mode"=FALSE, "axis 1: \nTarget GND"=FALSE, "axis 2: \nTarget GND"=FALSE, "Set static Amplitude when moving?"=FALSE, "Static Amplitude (mV)"=0.0} ("Inputs"), "Axes Number"=w101, "Axis 1: sp Position"="axis 1:\nsp rot count", "Axis 1: sp rot count"="axis 1:\nsp position °", "Set static Amplitude when moving?"="set static amplitude\nwhen moving", "Static Amplitude (mV)"=w97) -> (w106:T2)
                n39 = call "To JSON Text.vim"("Anything"=w106) -> ("<JSON>"=w105:string)  [unwired: 9 in, 1 out]
                n40 = Bundle By Name(cluster=w103, "Message.Command"="StaticAmplitude\nMoveAbsolute", "Message.Data"=w105) -> (w104:T10)
                n41 = call <vilib>:"Add State(s) to Queue__jki_lib_state_machine.vi"("State(s) in Front (\"\")"="Data: Set UI Cluster\nData: Set Config Cluster\nAction: Send Message to Instrument\nAction: getAll\nUI: Update FP Indicators" ("State(s) in Front (\"\")"), "State(s) in (\"\")"=w111) -> ("States Out"=w110:string)  [unwired: 13 in]
              }
              event "axis 2:\nAbsolute": Value Change {
                w113 = 1000.0 ("static amplitude (mV)")
                w117 = u8 1 items=["1", "2", "3", "4", "5", "6", "7", "8", "9"] ("axis no")
                n42 = event-data() -> ("OldVal"=w114:bool)  [unwired: 1 in, 5 out]
                n43 = local write "static amplitude (mV)"(w113) -> ()
                n44 = local write "axis 2:\nAbsolute"(w114) -> ()
                n45 = local read "set static amplitude\nwhen moving"() -> (w112:bool)
                n46 = Bundle By Name(cluster=T2 {"Handle"=0, "Axes Number"=0, "Axis 1: sp Position"=0.0, "Axis 2: sp Position"=0.0, "Axis 1: sp rot count"=0, "Axis 2: sp rot count"=0, "Backward or Forward?"=FALSE, "Axis 1: Amplitude [V] "=0.0, "Axis 2: Amplitude [V] "=0.0, "Axis 1: DCLevel [V]"=0.0, "Axis 2: DCLevel [V]"=0.0, "Axis 1: Frequency [Hz]"=0, "Axis 2: Frequency [Hz]"=0, "Axis 1:\ncontrol mode"=enum."amplitude", "Axis 2:\ncontrol mode"=enum."amplitude", "axis 1:\nOutput"=FALSE, "axis 2:\nOutput 2"=FALSE, "axis 1:\nstop detection"=FALSE, "axis 2:\nstop detection"=FALSE, "axis 1:\nSingle Circle Mode"=FALSE, "axis 2:\nSingle Circle Mode"=FALSE, "axis 1: \nTarget GND"=FALSE, "axis 2: \nTarget GND"=FALSE, "Set static Amplitude when moving?"=FALSE, "Static Amplitude (mV)"=0.0} ("Inputs"), "Axes Number"=w117, "Axis 2: sp Position"="axis 2:\nsp position °", "Axis 2: sp rot count"="axis 2:\nsp rot count", "Set static Amplitude when moving?"=w112, "Static Amplitude (mV)"=w113) -> (w122:T2)
                n47 = call "To JSON Text.vim"("Anything"=w122) -> ("<JSON>"=w121:string)  [unwired: 9 in, 1 out]
                n48 = Bundle By Name(cluster=w119, "Message.Command"="StaticAmplitude\nMoveAbsolute", "Message.Data"=w121) -> (w120:T10)
                n49 = call <vilib>:"Add State(s) to Queue__jki_lib_state_machine.vi"("State(s) in Front (\"\")"="Data: Set UI Cluster\nData: Set Config Cluster\nAction: Send Message to Instrument\nAction: getAll\nUI: Update FP Indicators" ("State(s) in Front (\"\")"), "State(s) in (\"\")"=w127) -> ("States Out"=w126:string)  [unwired: 13 in]
              }
              event "axis 1:\nRelative": Value Change {
                w131 = u8 0 items=["1", "2", "3", "4", "5", "6", "7", "8", "9"] ("axis no")
                n50 = event-data() -> ("OldVal"=w130:bool)  [unwired: 1 in, 5 out]
                n51 = local read "axis 1:\nsp rot count"() -> (w128:i32)
                n52 = local read "axis 1:\nsp position °"() -> (w129:dbl)
                n53 = local write "axis 1:\nRelative"(w130) -> ()
                n54 = Bundle By Name(cluster=T2 {"Handle"=0, "Axes Number"=0, "Axis 1: sp Position"=0.0, "Axis 2: sp Position"=0.0, "Axis 1: sp rot count"=0, "Axis 2: sp rot count"=0, "Backward or Forward?"=FALSE, "Axis 1: Amplitude [V] "=0.0, "Axis 2: Amplitude [V] "=0.0, "Axis 1: DCLevel [V]"=0.0, "Axis 2: DCLevel [V]"=0.0, "Axis 1: Frequency [Hz]"=0, "Axis 2: Frequency [Hz]"=0, "Axis 1:\ncontrol mode"=enum."amplitude", "Axis 2:\ncontrol mode"=enum."amplitude", "axis 1:\nOutput"=FALSE, "axis 2:\nOutput 2"=FALSE, "axis 1:\nstop detection"=FALSE, "axis 2:\nstop detection"=FALSE, "axis 1:\nSingle Circle Mode"=FALSE, "axis 2:\nSingle Circle Mode"=FALSE, "axis 1: \nTarget GND"=FALSE, "axis 2: \nTarget GND"=FALSE, "Set static Amplitude when moving?"=FALSE, "Static Amplitude (mV)"=0.0} ("Inputs"), "Axes Number"=w131, "Axis 1: sp Position"=w128, "Axis 1: sp rot count"=w129) -> (w136:T2)
                n55 = call "To JSON Text.vim"("Anything"=w136) -> ("<JSON>"=w135:string)  [unwired: 9 in, 1 out]
                n56 = Bundle By Name(cluster=w133, "Message.Command"="MoveRelative", "Message.Data"=w135) -> (w134:T10)
                n57 = call <vilib>:"Add State(s) to Queue__jki_lib_state_machine.vi"("State(s) in Front (\"\")"="Data: Set UI Cluster\nData: Set Config Cluster\nAction: Send Message to Instrument\nAction: getAll\nUI: Update FP Indicators" ("State(s) in Front (\"\")"), "State(s) in (\"\")"=w141) -> ("States Out"=w140:string)  [unwired: 13 in]
              }
              event "axis 2:\nRelative": Value Change {
                w145 = u8 1 items=["1", "2", "3", "4", "5", "6", "7", "8", "9"] ("axis no")
                n58 = event-data() -> ("OldVal"=w144:bool)  [unwired: 1 in, 5 out]
                n59 = local read "axis 2:\nsp position °"() -> (w142:i32)
                n60 = local read "axis 2:\nsp rot count"() -> (w143:dbl)
                n61 = local write "axis 2:\nRelative"(w144) -> ()
                n62 = Bundle By Name(cluster=T2 {"Handle"=0, "Axes Number"=0, "Axis 1: sp Position"=0.0, "Axis 2: sp Position"=0.0, "Axis 1: sp rot count"=0, "Axis 2: sp rot count"=0, "Backward or Forward?"=FALSE, "Axis 1: Amplitude [V] "=0.0, "Axis 2: Amplitude [V] "=0.0, "Axis 1: DCLevel [V]"=0.0, "Axis 2: DCLevel [V]"=0.0, "Axis 1: Frequency [Hz]"=0, "Axis 2: Frequency [Hz]"=0, "Axis 1:\ncontrol mode"=enum."amplitude", "Axis 2:\ncontrol mode"=enum."amplitude", "axis 1:\nOutput"=FALSE, "axis 2:\nOutput 2"=FALSE, "axis 1:\nstop detection"=FALSE, "axis 2:\nstop detection"=FALSE, "axis 1:\nSingle Circle Mode"=FALSE, "axis 2:\nSingle Circle Mode"=FALSE, "axis 1: \nTarget GND"=FALSE, "axis 2: \nTarget GND"=FALSE, "Set static Amplitude when moving?"=FALSE, "Static Amplitude (mV)"=0.0} ("Inputs"), "Axes Number"=w145, "Axis 2: sp Position"=w142, "Axis 2: sp rot count"=w143) -> (w150:T2)
                n63 = call "To JSON Text.vim"("Anything"=w150) -> ("<JSON>"=w149:string)  [unwired: 9 in, 1 out]
                n64 = Bundle By Name(cluster=w147, "Message.Command"="MoveRelative", "Message.Data"=w149) -> (w148:T10)
                n65 = call <vilib>:"Add State(s) to Queue__jki_lib_state_machine.vi"("State(s) in Front (\"\")"="Data: Set UI Cluster\nData: Set Config Cluster\nAction: Send Message to Instrument\nAction: getAll\nUI: Update FP Indicators" ("State(s) in Front (\"\")"), "State(s) in (\"\")"=w155) -> ("States Out"=w154:string)  [unwired: 13 in]
              }
              event "axis 1:\nsingle step fwd": Value Change {
                w157 = u8 0 items=["1", "2", "3", "4", "5", "6", "7", "8", "9"] ("axis no")
                n66 = event-data() -> ()  [unwired: 1 in, 6 out]
                n67 = Bundle By Name(cluster=T2 {"Handle"=0, "Axes Number"=0, "Axis 1: sp Position"=0.0, "Axis 2: sp Position"=0.0, "Axis 1: sp rot count"=0, "Axis 2: sp rot count"=0, "Backward or Forward?"=FALSE, "Axis 1: Amplitude [V] "=0.0, "Axis 2: Amplitude [V] "=0.0, "Axis 1: DCLevel [V]"=0.0, "Axis 2: DCLevel [V]"=0.0, "Axis 1: Frequency [Hz]"=0, "Axis 2: Frequency [Hz]"=0, "Axis 1:\ncontrol mode"=enum."amplitude", "Axis 2:\ncontrol mode"=enum."amplitude", "axis 1:\nOutput"=FALSE, "axis 2:\nOutput 2"=FALSE, "axis 1:\nstop detection"=FALSE, "axis 2:\nstop detection"=FALSE, "axis 1:\nSingle Circle Mode"=FALSE, "axis 2:\nSingle Circle Mode"=FALSE, "axis 1: \nTarget GND"=FALSE, "axis 2: \nTarget GND"=FALSE, "Set static Amplitude when moving?"=FALSE, "Static Amplitude (mV)"=0.0} ("Inputs"), "Axes Number"=w157, "Backward or Forward?"=FALSE ("Backward or Farward?")) -> (w162:T2)
                n68 = call "To JSON Text.vim"("Anything"=w162) -> ("<JSON>"=w161:string)  [unwired: 9 in, 1 out]
                n69 = Bundle By Name(cluster=w159, "Message.Command"="MoveSingleStep", "Message.Data"=w161) -> (w160:T10)
                n70 = call <vilib>:"Add State(s) to Queue__jki_lib_state_machine.vi"("State(s) in Front (\"\")"="Data: Set UI Cluster\nData: Set Config Cluster\nAction: Send Message to Instrument\nAction: getAll\nUI: Update FP Indicators" ("State(s) in Front (\"\")"), "State(s) in (\"\")"=w167) -> ("States Out"=w166:string)  [unwired: 13 in]
              }
              event "axis 2:\nsingle step fwd": Value Change {
                w169 = u8 1 items=["1", "2", "3", "4", "5", "6", "7", "8", "9"] ("axis no")
                n71 = event-data() -> ()  [unwired: 1 in, 6 out]
                n72 = Bundle By Name(cluster=T2 {"Handle"=0, "Axes Number"=0, "Axis 1: sp Position"=0.0, "Axis 2: sp Position"=0.0, "Axis 1: sp rot count"=0, "Axis 2: sp rot count"=0, "Backward or Forward?"=FALSE, "Axis 1: Amplitude [V] "=0.0, "Axis 2: Amplitude [V] "=0.0, "Axis 1: DCLevel [V]"=0.0, "Axis 2: DCLevel [V]"=0.0, "Axis 1: Frequency [Hz]"=0, "Axis 2: Frequency [Hz]"=0, "Axis 1:\ncontrol mode"=enum."amplitude", "Axis 2:\ncontrol mode"=enum."amplitude", "axis 1:\nOutput"=FALSE, "axis 2:\nOutput 2"=FALSE, "axis 1:\nstop detection"=FALSE, "axis 2:\nstop detection"=FALSE, "axis 1:\nSingle Circle Mode"=FALSE, "axis 2:\nSingle Circle Mode"=FALSE, "axis 1: \nTarget GND"=FALSE, "axis 2: \nTarget GND"=FALSE, "Set static Amplitude when moving?"=FALSE, "Static Amplitude (mV)"=0.0} ("Inputs"), "Axes Number"=w169, "Backward or Forward?"=FALSE ("Backward or Farward?")) -> (w174:T2)
                n73 = call "To JSON Text.vim"("Anything"=w174) -> ("<JSON>"=w173:string)  [unwired: 9 in, 1 out]
                n74 = Bundle By Name(cluster=w171, "Message.Command"="MoveSingleStep", "Message.Data"=w173) -> (w172:T10)
                n75 = call <vilib>:"Add State(s) to Queue__jki_lib_state_machine.vi"("State(s) in Front (\"\")"="Data: Set UI Cluster\nData: Set Config Cluster\nAction: Send Message to Instrument\nAction: getAll\nUI: Update FP Indicators" ("State(s) in Front (\"\")"), "State(s) in (\"\")"=w179) -> ("States Out"=w178:string)  [unwired: 13 in]
              }
              event "axis 1:\nsingle step back": Value Change {
                w181 = u8 0 items=["1", "2", "3", "4", "5", "6", "7", "8", "9"] ("axis no")
                n76 = event-data() -> ()  [unwired: 1 in, 6 out]
                n77 = Bundle By Name(cluster=T2 {"Handle"=0, "Axes Number"=0, "Axis 1: sp Position"=0.0, "Axis 2: sp Position"=0.0, "Axis 1: sp rot count"=0, "Axis 2: sp rot count"=0, "Backward or Forward?"=FALSE, "Axis 1: Amplitude [V] "=0.0, "Axis 2: Amplitude [V] "=0.0, "Axis 1: DCLevel [V]"=0.0, "Axis 2: DCLevel [V]"=0.0, "Axis 1: Frequency [Hz]"=0, "Axis 2: Frequency [Hz]"=0, "Axis 1:\ncontrol mode"=enum."amplitude", "Axis 2:\ncontrol mode"=enum."amplitude", "axis 1:\nOutput"=FALSE, "axis 2:\nOutput 2"=FALSE, "axis 1:\nstop detection"=FALSE, "axis 2:\nstop detection"=FALSE, "axis 1:\nSingle Circle Mode"=FALSE, "axis 2:\nSingle Circle Mode"=FALSE, "axis 1: \nTarget GND"=FALSE, "axis 2: \nTarget GND"=FALSE, "Set static Amplitude when moving?"=FALSE, "Static Amplitude (mV)"=0.0} ("Inputs"), "Axes Number"=w181, "Backward or Forward?"=TRUE ("Backward or Farward?")) -> (w186:T2)
                n78 = call "To JSON Text.vim"("Anything"=w186) -> ("<JSON>"=w185:string)  [unwired: 9 in, 1 out]
                n79 = Bundle By Name(cluster=w183, "Message.Command"="MoveSingleStep", "Message.Data"=w185) -> (w184:T10)
                n80 = call <vilib>:"Add State(s) to Queue__jki_lib_state_machine.vi"("State(s) in Front (\"\")"="Data: Set UI Cluster\nData: Set Config Cluster\nAction: Send Message to Instrument\nAction: getAll\nUI: Update FP Indicators" ("State(s) in Front (\"\")"), "State(s) in (\"\")"=w191) -> ("States Out"=w190:string)  [unwired: 13 in]
              }
              event "axis 2:\nsingle step back": Value Change {
                w193 = u8 1 items=["1", "2", "3", "4", "5", "6", "7", "8", "9"] ("axis no")
                n81 = event-data() -> ()  [unwired: 1 in, 6 out]
                n82 = Bundle By Name(cluster=T2 {"Handle"=0, "Axes Number"=0, "Axis 1: sp Position"=0.0, "Axis 2: sp Position"=0.0, "Axis 1: sp rot count"=0, "Axis 2: sp rot count"=0, "Backward or Forward?"=FALSE, "Axis 1: Amplitude [V] "=0.0, "Axis 2: Amplitude [V] "=0.0, "Axis 1: DCLevel [V]"=0.0, "Axis 2: DCLevel [V]"=0.0, "Axis 1: Frequency [Hz]"=0, "Axis 2: Frequency [Hz]"=0, "Axis 1:\ncontrol mode"=enum."amplitude", "Axis 2:\ncontrol mode"=enum."amplitude", "axis 1:\nOutput"=FALSE, "axis 2:\nOutput 2"=FALSE, "axis 1:\nstop detection"=FALSE, "axis 2:\nstop detection"=FALSE, "axis 1:\nSingle Circle Mode"=FALSE, "axis 2:\nSingle Circle Mode"=FALSE, "axis 1: \nTarget GND"=FALSE, "axis 2: \nTarget GND"=FALSE, "Set static Amplitude when moving?"=FALSE, "Static Amplitude (mV)"=0.0} ("Inputs"), "Axes Number"=w193, "Backward or Forward?"=TRUE ("Backward or Farward?")) -> (w198:T2)
                n83 = call "To JSON Text.vim"("Anything"=w198) -> ("<JSON>"=w197:string)  [unwired: 9 in, 1 out]
                n84 = Bundle By Name(cluster=w195, "Message.Command"="MoveSingleStep", "Message.Data"=w197) -> (w196:T10)
                n85 = call <vilib>:"Add State(s) to Queue__jki_lib_state_machine.vi"("State(s) in Front (\"\")"="Data: Set UI Cluster\nData: Set Config Cluster\nAction: Send Message to Instrument\nAction: getAll\nUI: Update FP Indicators" ("State(s) in Front (\"\")"), "State(s) in (\"\")"=w203) -> ("States Out"=w202:string)  [unwired: 13 in]
              }
              event "axis 1:\ncontinuous fwd": Value Change {
                n86 = event-data() -> ()  [unwired: 1 in, 6 out]
                n87 = case shown="False" "axis 1:\ncontinuous fwd" {
                  tunnel: [w211 w222] -> w206
                  tunnel: w205 -> [w212 w221]
                  frame False {
                    w213 = u8 0 items=["1", "2", "3", "4", "5", "6", "7", "8", "9"] ("axis no")
                    n88 = Bundle By Name(cluster=T2 {"Handle"=0, "Axes Number"=0, "Axis 1: sp Position"=0.0, "Axis 2: sp Position"=0.0, "Axis 1: sp rot count"=0, "Axis 2: sp rot count"=0, "Backward or Forward?"=FALSE, "Axis 1: Amplitude [V] "=0.0, "Axis 2: Amplitude [V] "=0.0, "Axis 1: DCLevel [V]"=0.0, "Axis 2: DCLevel [V]"=0.0, "Axis 1: Frequency [Hz]"=0, "Axis 2: Frequency [Hz]"=0, "Axis 1:\ncontrol mode"=enum."amplitude", "Axis 2:\ncontrol mode"=enum."amplitude", "axis 1:\nOutput"=FALSE, "axis 2:\nOutput 2"=FALSE, "axis 1:\nstop detection"=FALSE, "axis 2:\nstop detection"=FALSE, "axis 1:\nSingle Circle Mode"=FALSE, "axis 2:\nSingle Circle Mode"=FALSE, "axis 1: \nTarget GND"=FALSE, "axis 2: \nTarget GND"=FALSE, "Set static Amplitude when moving?"=FALSE, "Static Amplitude (mV)"=0.0} ("Inputs"), "Axes Number"=w213) -> (w216:T2)
                    n89 = call "To JSON Text.vim"("Anything"=w216) -> ("<JSON>"=w215:string)  [unwired: 9 in, 1 out]
                    n90 = Bundle By Name(cluster=w212, "Message.Command"="StopMoving", "Message.Data"=w215) -> (w211:T10)
                  }
                  frame True {
                    w219 = u8 0 items=["1", "2", "3", "4", "5", "6", "7", "8", "9"] ("axis no")
                    n91 = Bundle By Name(cluster=T2 {"Handle"=0, "Axes Number"=0, "Axis 1: sp Position"=0.0, "Axis 2: sp Position"=0.0, "Axis 1: sp rot count"=0, "Axis 2: sp rot count"=0, "Backward or Forward?"=FALSE, "Axis 1: Amplitude [V] "=0.0, "Axis 2: Amplitude [V] "=0.0, "Axis 1: DCLevel [V]"=0.0, "Axis 2: DCLevel [V]"=0.0, "Axis 1: Frequency [Hz]"=0, "Axis 2: Frequency [Hz]"=0, "Axis 1:\ncontrol mode"=enum."amplitude", "Axis 2:\ncontrol mode"=enum."amplitude", "axis 1:\nOutput"=FALSE, "axis 2:\nOutput 2"=FALSE, "axis 1:\nstop detection"=FALSE, "axis 2:\nstop detection"=FALSE, "axis 1:\nSingle Circle Mode"=FALSE, "axis 2:\nSingle Circle Mode"=FALSE, "axis 1: \nTarget GND"=FALSE, "axis 2: \nTarget GND"=FALSE, "Set static Amplitude when moving?"=FALSE, "Static Amplitude (mV)"=0.0} ("Inputs"), "Axes Number"=w219, "Backward or Forward?"=FALSE ("Backward or Farward?")) -> (w224:T2)
                    n92 = call "To JSON Text.vim"("Anything"=w224) -> ("<JSON>"=w223:string)  [unwired: 9 in, 1 out]
                    n93 = Bundle By Name(cluster=w221, "Message.Command"="MoveContinuous", "Message.Data"=w223) -> (w222:T10)
                  }
                }
                n94 = call <vilib>:"Add State(s) to Queue__jki_lib_state_machine.vi"("State(s) in Front (\"\")"="Data: Set UI Cluster\nData: Set Config Cluster\nAction: Send Message to Instrument\nAction: getAll\nUI: Update FP Indicators" ("State(s) in Front (\"\")"), "State(s) in (\"\")"=w210) -> ("States Out"=w209:string)  [unwired: 13 in]
              }
              event "axis 2:\ncontinuous fwd": Value Change {
                n95 = event-data() -> ()  [unwired: 1 in, 6 out]
                n96 = case shown="False" "axis 2:\ncontinuous fwd" {
                  tunnel: [w233 w244] -> w228
                  tunnel: w227 -> [w234 w243]
                  frame False {
                    w235 = u8 1 items=["1", "2", "3", "4", "5", "6", "7", "8", "9"] ("axis no")
                    n97 = Bundle By Name(cluster=T2 {"Handle"=0, "Axes Number"=0, "Axis 1: sp Position"=0.0, "Axis 2: sp Position"=0.0, "Axis 1: sp rot count"=0, "Axis 2: sp rot count"=0, "Backward or Forward?"=FALSE, "Axis 1: Amplitude [V] "=0.0, "Axis 2: Amplitude [V] "=0.0, "Axis 1: DCLevel [V]"=0.0, "Axis 2: DCLevel [V]"=0.0, "Axis 1: Frequency [Hz]"=0, "Axis 2: Frequency [Hz]"=0, "Axis 1:\ncontrol mode"=enum."amplitude", "Axis 2:\ncontrol mode"=enum."amplitude", "axis 1:\nOutput"=FALSE, "axis 2:\nOutput 2"=FALSE, "axis 1:\nstop detection"=FALSE, "axis 2:\nstop detection"=FALSE, "axis 1:\nSingle Circle Mode"=FALSE, "axis 2:\nSingle Circle Mode"=FALSE, "axis 1: \nTarget GND"=FALSE, "axis 2: \nTarget GND"=FALSE, "Set static Amplitude when moving?"=FALSE, "Static Amplitude (mV)"=0.0} ("Inputs"), "Axes Number"=w235) -> (w238:T2)
                    n98 = call "To JSON Text.vim"("Anything"=w238) -> ("<JSON>"=w237:string)  [unwired: 9 in, 1 out]
                    n99 = Bundle By Name(cluster=w234, "Message.Command"="StopMoving", "Message.Data"=w237) -> (w233:T10)
                  }
                  frame True {
                    w241 = u8 1 items=["1", "2", "3", "4", "5", "6", "7", "8", "9"] ("axis no")
                    n100 = Bundle By Name(cluster=T2 {"Handle"=0, "Axes Number"=0, "Axis 1: sp Position"=0.0, "Axis 2: sp Position"=0.0, "Axis 1: sp rot count"=0, "Axis 2: sp rot count"=0, "Backward or Forward?"=FALSE, "Axis 1: Amplitude [V] "=0.0, "Axis 2: Amplitude [V] "=0.0, "Axis 1: DCLevel [V]"=0.0, "Axis 2: DCLevel [V]"=0.0, "Axis 1: Frequency [Hz]"=0, "Axis 2: Frequency [Hz]"=0, "Axis 1:\ncontrol mode"=enum."amplitude", "Axis 2:\ncontrol mode"=enum."amplitude", "axis 1:\nOutput"=FALSE, "axis 2:\nOutput 2"=FALSE, "axis 1:\nstop detection"=FALSE, "axis 2:\nstop detection"=FALSE, "axis 1:\nSingle Circle Mode"=FALSE, "axis 2:\nSingle Circle Mode"=FALSE, "axis 1: \nTarget GND"=FALSE, "axis 2: \nTarget GND"=FALSE, "Set static Amplitude when moving?"=FALSE, "Static Amplitude (mV)"=0.0} ("Inputs"), "Axes Number"=w241, "Backward or Forward?"=FALSE ("Backward or Farward?")) -> (w246:T2)
                    n101 = call "To JSON Text.vim"("Anything"=w246) -> ("<JSON>"=w245:string)  [unwired: 9 in, 1 out]
                    n102 = Bundle By Name(cluster=w243, "Message.Command"="MoveContinuous", "Message.Data"=w245) -> (w244:T10)
                  }
                }
                n103 = call <vilib>:"Add State(s) to Queue__jki_lib_state_machine.vi"("State(s) in Front (\"\")"="Data: Set UI Cluster\nData: Set Config Cluster\nAction: Send Message to Instrument\nAction: getAll\nUI: Update FP Indicators" ("State(s) in Front (\"\")"), "State(s) in (\"\")"=w232) -> ("States Out"=w231:string)  [unwired: 13 in]
              }
              event "axis 1:\ncontinuous back": Value Change {
                n104 = event-data() -> ()  [unwired: 1 in, 6 out]
                n105 = case shown="False" "axis 1:\ncontinuous back" {
                  tunnel: [w255 w266] -> w250
                  tunnel: w249 -> [w256 w265]
                  frame False {
                    w257 = u8 0 items=["1", "2", "3", "4", "5", "6", "7", "8", "9"] ("axis no")
                    n106 = Bundle By Name(cluster=T2 {"Handle"=0, "Axes Number"=0, "Axis 1: sp Position"=0.0, "Axis 2: sp Position"=0.0, "Axis 1: sp rot count"=0, "Axis 2: sp rot count"=0, "Backward or Forward?"=FALSE, "Axis 1: Amplitude [V] "=0.0, "Axis 2: Amplitude [V] "=0.0, "Axis 1: DCLevel [V]"=0.0, "Axis 2: DCLevel [V]"=0.0, "Axis 1: Frequency [Hz]"=0, "Axis 2: Frequency [Hz]"=0, "Axis 1:\ncontrol mode"=enum."amplitude", "Axis 2:\ncontrol mode"=enum."amplitude", "axis 1:\nOutput"=FALSE, "axis 2:\nOutput 2"=FALSE, "axis 1:\nstop detection"=FALSE, "axis 2:\nstop detection"=FALSE, "axis 1:\nSingle Circle Mode"=FALSE, "axis 2:\nSingle Circle Mode"=FALSE, "axis 1: \nTarget GND"=FALSE, "axis 2: \nTarget GND"=FALSE, "Set static Amplitude when moving?"=FALSE, "Static Amplitude (mV)"=0.0} ("Inputs"), "Axes Number"=w257) -> (w260:T2)
                    n107 = call "To JSON Text.vim"("Anything"=w260) -> ("<JSON>"=w259:string)  [unwired: 9 in, 1 out]
                    n108 = Bundle By Name(cluster=w256, "Message.Command"="StopMoving", "Message.Data"=w259) -> (w255:T10)
                  }
                  frame True {
                    w263 = u8 0 items=["1", "2", "3", "4", "5", "6", "7", "8", "9"] ("axis no")
                    n109 = Bundle By Name(cluster=T2 {"Handle"=0, "Axes Number"=0, "Axis 1: sp Position"=0.0, "Axis 2: sp Position"=0.0, "Axis 1: sp rot count"=0, "Axis 2: sp rot count"=0, "Backward or Forward?"=FALSE, "Axis 1: Amplitude [V] "=0.0, "Axis 2: Amplitude [V] "=0.0, "Axis 1: DCLevel [V]"=0.0, "Axis 2: DCLevel [V]"=0.0, "Axis 1: Frequency [Hz]"=0, "Axis 2: Frequency [Hz]"=0, "Axis 1:\ncontrol mode"=enum."amplitude", "Axis 2:\ncontrol mode"=enum."amplitude", "axis 1:\nOutput"=FALSE, "axis 2:\nOutput 2"=FALSE, "axis 1:\nstop detection"=FALSE, "axis 2:\nstop detection"=FALSE, "axis 1:\nSingle Circle Mode"=FALSE, "axis 2:\nSingle Circle Mode"=FALSE, "axis 1: \nTarget GND"=FALSE, "axis 2: \nTarget GND"=FALSE, "Set static Amplitude when moving?"=FALSE, "Static Amplitude (mV)"=0.0} ("Inputs"), "Axes Number"=w263, "Backward or Forward?"=FALSE ("Backward or Farward?")) -> (w268:T2)
                    n110 = call "To JSON Text.vim"("Anything"=w268) -> ("<JSON>"=w267:string)  [unwired: 9 in, 1 out]
                    n111 = Bundle By Name(cluster=w265, "Message.Command"="MoveContinuous", "Message.Data"=w267) -> (w266:T10)
                  }
                }
                n112 = call <vilib>:"Add State(s) to Queue__jki_lib_state_machine.vi"("State(s) in Front (\"\")"="Data: Set UI Cluster\nData: Set Config Cluster\nAction: Send Message to Instrument\nAction: getAll\nUI: Update FP Indicators" ("State(s) in Front (\"\")"), "State(s) in (\"\")"=w254) -> ("States Out"=w253:string)  [unwired: 13 in]
              }
              event "axis 2:\ncontinuous back": Value Change {
                n113 = event-data() -> ()  [unwired: 1 in, 6 out]
                n114 = case shown="False" "axis 2:\ncontinuous back" {
                  tunnel: [w277 w289] -> w272
                  tunnel: w271 -> [w278 w288]
                  frame False {
                    w279 = u8 1 items=["1", "2", "3", "4", "5", "6", "7", "8", "9"] ("axis no")
                    n115 = Bundle By Name(cluster=T2 {"Handle"=0, "Axes Number"=0, "Axis 1: sp Position"=0.0, "Axis 2: sp Position"=0.0, "Axis 1: sp rot count"=0, "Axis 2: sp rot count"=0, "Backward or Forward?"=FALSE, "Axis 1: Amplitude [V] "=0.0, "Axis 2: Amplitude [V] "=0.0, "Axis 1: DCLevel [V]"=0.0, "Axis 2: DCLevel [V]"=0.0, "Axis 1: Frequency [Hz]"=0, "Axis 2: Frequency [Hz]"=0, "Axis 1:\ncontrol mode"=enum."amplitude", "Axis 2:\ncontrol mode"=enum."amplitude", "axis 1:\nOutput"=FALSE, "axis 2:\nOutput 2"=FALSE, "axis 1:\nstop detection"=FALSE, "axis 2:\nstop detection"=FALSE, "axis 1:\nSingle Circle Mode"=FALSE, "axis 2:\nSingle Circle Mode"=FALSE, "axis 1: \nTarget GND"=FALSE, "axis 2: \nTarget GND"=FALSE, "Set static Amplitude when moving?"=FALSE, "Static Amplitude (mV)"=0.0} ("Inputs"), "Axes Number"=w279) -> (w282:T2)
                    n116 = call "To JSON Text.vim"("Anything"=w282) -> ("<JSON>"=w281:string)  [unwired: 9 in, 1 out]
                    n117 = Bundle By Name(cluster=w278, "Message.Command"="StopMoving", "Message.Data"=w281) -> (w277:T10)
                  }
                  frame True {
                    w286 = u8 1 items=["1", "2", "3", "4", "5", "6", "7", "8", "9"] ("axis no")
                    n118 = Bundle By Name(cluster=T2 {"Handle"=0, "Axes Number"=0, "Axis 1: sp Position"=0.0, "Axis 2: sp Position"=0.0, "Axis 1: sp rot count"=0, "Axis 2: sp rot count"=0, "Backward or Forward?"=FALSE, "Axis 1: Amplitude [V] "=0.0, "Axis 2: Amplitude [V] "=0.0, "Axis 1: DCLevel [V]"=0.0, "Axis 2: DCLevel [V]"=0.0, "Axis 1: Frequency [Hz]"=0, "Axis 2: Frequency [Hz]"=0, "Axis 1:\ncontrol mode"=enum."amplitude", "Axis 2:\ncontrol mode"=enum."amplitude", "axis 1:\nOutput"=FALSE, "axis 2:\nOutput 2"=FALSE, "axis 1:\nstop detection"=FALSE, "axis 2:\nstop detection"=FALSE, "axis 1:\nSingle Circle Mode"=FALSE, "axis 2:\nSingle Circle Mode"=FALSE, "axis 1: \nTarget GND"=FALSE, "axis 2: \nTarget GND"=FALSE, "Set static Amplitude when moving?"=FALSE, "Static Amplitude (mV)"=0.0} ("Inputs"), "Axes Number"=w286, "Backward or Forward?"=TRUE ("Backward or Farward?")) -> (w290:T2)
                    n119 = call "To JSON Text.vim"("Anything"=w290) -> ("<JSON>"=w284:string)  [unwired: 9 in, 1 out]
                    n120 = Bundle By Name(cluster=w288, "Message.Command"="MoveContinuous", "Message.Data"=w284) -> (w289:T10)
                  }
                }
                n121 = call <vilib>:"Add State(s) to Queue__jki_lib_state_machine.vi"("State(s) in Front (\"\")"="Data: Set UI Cluster\nData: Set Config Cluster\nAction: Send Message to Instrument\nAction: getAll\nUI: Update FP Indicators" ("State(s) in Front (\"\")"), "State(s) in (\"\")"=w276) -> ("States Out"=w275:string)  [unwired: 13 in]
              }
              event "axis 2:\nAmplitude [V]": Value Change {
                w293 = u8 1 items=["1", "2", "3", "4", "5", "6", "7", "8", "9"] ("axis no")
                n122 = event-data() -> ()  [unwired: 1 in, 6 out]
                n123 = Bundle By Name(cluster=T2 {"Handle"=0, "Axes Number"=0, "Axis 1: sp Position"=0.0, "Axis 2: sp Position"=0.0, "Axis 1: sp rot count"=0, "Axis 2: sp rot count"=0, "Backward or Forward?"=FALSE, "Axis 1: Amplitude [V] "=0.0, "Axis 2: Amplitude [V] "=0.0, "Axis 1: DCLevel [V]"=0.0, "Axis 2: DCLevel [V]"=0.0, "Axis 1: Frequency [Hz]"=0, "Axis 2: Frequency [Hz]"=0, "Axis 1:\ncontrol mode"=enum."amplitude", "Axis 2:\ncontrol mode"=enum."amplitude", "axis 1:\nOutput"=FALSE, "axis 2:\nOutput 2"=FALSE, "axis 1:\nstop detection"=FALSE, "axis 2:\nstop detection"=FALSE, "axis 1:\nSingle Circle Mode"=FALSE, "axis 2:\nSingle Circle Mode"=FALSE, "axis 1: \nTarget GND"=FALSE, "axis 2: \nTarget GND"=FALSE, "Set static Amplitude when moving?"=FALSE, "Static Amplitude (mV)"=0.0} ("Inputs"), "Axes Number"=w293, "Axis 2: Amplitude [V]"="axis 2:\nAmplitude [V]") -> (w298:T2)
                n124 = call "To JSON Text.vim"("Anything"=w298) -> ("<JSON>"=w297:string)  [unwired: 9 in, 1 out]
                n125 = Bundle By Name(cluster=w295, "Message.Command"="Amplitude", "Message.Data"=w297) -> (w296:T10)
                n126 = call <vilib>:"Add State(s) to Queue__jki_lib_state_machine.vi"("State(s) in Front (\"\")"="Data: Set UI Cluster\nData: Set Config Cluster\nAction: Send Message to Instrument\nAction: getAll\nUI: Update FP Indicators" ("State(s) in Front (\"\")"), "State(s) in (\"\")"=w303) -> ("States Out"=w302:string)  [unwired: 13 in]
              }
              event "axis 1:\nAmplitude [V]": Value Change {
                w305 = u8 0 items=["1", "2", "3", "4", "5", "6", "7", "8", "9"] ("axis no")
                n127 = event-data() -> ()  [unwired: 1 in, 6 out]
                n128 = Bundle By Name(cluster=T2 {"Handle"=0, "Axes Number"=0, "Axis 1: sp Position"=0.0, "Axis 2: sp Position"=0.0, "Axis 1: sp rot count"=0, "Axis 2: sp rot count"=0, "Backward or Forward?"=FALSE, "Axis 1: Amplitude [V] "=0.0, "Axis 2: Amplitude [V] "=0.0, "Axis 1: DCLevel [V]"=0.0, "Axis 2: DCLevel [V]"=0.0, "Axis 1: Frequency [Hz]"=0, "Axis 2: Frequency [Hz]"=0, "Axis 1:\ncontrol mode"=enum."amplitude", "Axis 2:\ncontrol mode"=enum."amplitude", "axis 1:\nOutput"=FALSE, "axis 2:\nOutput 2"=FALSE, "axis 1:\nstop detection"=FALSE, "axis 2:\nstop detection"=FALSE, "axis 1:\nSingle Circle Mode"=FALSE, "axis 2:\nSingle Circle Mode"=FALSE, "axis 1: \nTarget GND"=FALSE, "axis 2: \nTarget GND"=FALSE, "Set static Amplitude when moving?"=FALSE, "Static Amplitude (mV)"=0.0} ("Inputs"), "Axes Number"=w305, "Axis 1: Amplitude [V]"="axis 1:\nAmplitude [V]") -> (w310:T2)
                n129 = call "To JSON Text.vim"("Anything"=w310) -> ("<JSON>"=w309:string)  [unwired: 9 in, 1 out]
                n130 = Bundle By Name(cluster=w307, "Message.Command"="Amplitude", "Message.Data"=w309) -> (w308:T10)
                n131 = call <vilib>:"Add State(s) to Queue__jki_lib_state_machine.vi"("State(s) in Front (\"\")"="Data: Set UI Cluster\nData: Set Config Cluster\nAction: Send Message to Instrument\nAction: getAll\nUI: Update FP Indicators" ("State(s) in Front (\"\")"), "State(s) in (\"\")"=w315) -> ("States Out"=w314:string)  [unwired: 13 in]
              }
              event "axis 1:\nDCLevel [V]": Value Change {
                w317 = u8 0 items=["1", "2", "3", "4", "5", "6", "7", "8", "9"] ("axis no")
                n132 = event-data() -> ()  [unwired: 1 in, 6 out]
                n133 = Bundle By Name(cluster=T2 {"Handle"=0, "Axes Number"=0, "Axis 1: sp Position"=0.0, "Axis 2: sp Position"=0.0, "Axis 1: sp rot count"=0, "Axis 2: sp rot count"=0, "Backward or Forward?"=FALSE, "Axis 1: Amplitude [V] "=0.0, "Axis 2: Amplitude [V] "=0.0, "Axis 1: DCLevel [V]"=0.0, "Axis 2: DCLevel [V]"=0.0, "Axis 1: Frequency [Hz]"=0, "Axis 2: Frequency [Hz]"=0, "Axis 1:\ncontrol mode"=enum."amplitude", "Axis 2:\ncontrol mode"=enum."amplitude", "axis 1:\nOutput"=FALSE, "axis 2:\nOutput 2"=FALSE, "axis 1:\nstop detection"=FALSE, "axis 2:\nstop detection"=FALSE, "axis 1:\nSingle Circle Mode"=FALSE, "axis 2:\nSingle Circle Mode"=FALSE, "axis 1: \nTarget GND"=FALSE, "axis 2: \nTarget GND"=FALSE, "Set static Amplitude when moving?"=FALSE, "Static Amplitude (mV)"=0.0} ("Inputs"), "Axes Number"=w317, "Axis 1: DCLevel [V]"="axis 1:\nDCLevel [V]") -> (w322:T2)
                n134 = call "To JSON Text.vim"("Anything"=w322) -> ("<JSON>"=w321:string)  [unwired: 9 in, 1 out]
                n135 = Bundle By Name(cluster=w319, "Message.Command"="DCLevel", "Message.Data"=w321) -> (w320:T10)
                n136 = call <vilib>:"Add State(s) to Queue__jki_lib_state_machine.vi"("State(s) in Front (\"\")"="Data: Set UI Cluster\nData: Set Config Cluster\nAction: Send Message to Instrument\nAction: getAll\nUI: Update FP Indicators" ("State(s) in Front (\"\")"), "State(s) in (\"\")"=w327) -> ("States Out"=w326:string)  [unwired: 13 in]
              }
              event "axis 2:\nDCLevel [V]": Value Change {
                w329 = u8 1 items=["1", "2", "3", "4", "5", "6", "7", "8", "9"] ("axis no")
                n137 = event-data() -> ()  [unwired: 1 in, 6 out]
                n138 = Bundle By Name(cluster=T2 {"Handle"=0, "Axes Number"=0, "Axis 1: sp Position"=0.0, "Axis 2: sp Position"=0.0, "Axis 1: sp rot count"=0, "Axis 2: sp rot count"=0, "Backward or Forward?"=FALSE, "Axis 1: Amplitude [V] "=0.0, "Axis 2: Amplitude [V] "=0.0, "Axis 1: DCLevel [V]"=0.0, "Axis 2: DCLevel [V]"=0.0, "Axis 1: Frequency [Hz]"=0, "Axis 2: Frequency [Hz]"=0, "Axis 1:\ncontrol mode"=enum."amplitude", "Axis 2:\ncontrol mode"=enum."amplitude", "axis 1:\nOutput"=FALSE, "axis 2:\nOutput 2"=FALSE, "axis 1:\nstop detection"=FALSE, "axis 2:\nstop detection"=FALSE, "axis 1:\nSingle Circle Mode"=FALSE, "axis 2:\nSingle Circle Mode"=FALSE, "axis 1: \nTarget GND"=FALSE, "axis 2: \nTarget GND"=FALSE, "Set static Amplitude when moving?"=FALSE, "Static Amplitude (mV)"=0.0} ("Inputs"), "Axes Number"=w329, "Axis 2: DCLevel [V]"="axis 2:\nDCLevel [V]") -> (w334:T2)
                n139 = call "To JSON Text.vim"("Anything"=w334) -> ("<JSON>"=w333:string)  [unwired: 9 in, 1 out]
                n140 = Bundle By Name(cluster=w331, "Message.Command"="DCLevel", "Message.Data"=w333) -> (w332:T10)
                n141 = call <vilib>:"Add State(s) to Queue__jki_lib_state_machine.vi"("State(s) in Front (\"\")"="Data: Set UI Cluster\nData: Set Config Cluster\nAction: Send Message to Instrument\nAction: getAll\nUI: Update FP Indicators" ("State(s) in Front (\"\")"), "State(s) in (\"\")"=w339) -> ("States Out"=w338:string)  [unwired: 13 in]
              }
              event "axis 1:\nFrequency [Hz]": Value Change {
                w341 = u8 0 items=["1", "2", "3", "4", "5", "6", "7", "8", "9"] ("axis no")
                n142 = event-data() -> ()  [unwired: 1 in, 6 out]
                n143 = Bundle By Name(cluster=T2 {"Handle"=0, "Axes Number"=0, "Axis 1: sp Position"=0.0, "Axis 2: sp Position"=0.0, "Axis 1: sp rot count"=0, "Axis 2: sp rot count"=0, "Backward or Forward?"=FALSE, "Axis 1: Amplitude [V] "=0.0, "Axis 2: Amplitude [V] "=0.0, "Axis 1: DCLevel [V]"=0.0, "Axis 2: DCLevel [V]"=0.0, "Axis 1: Frequency [Hz]"=0, "Axis 2: Frequency [Hz]"=0, "Axis 1:\ncontrol mode"=enum."amplitude", "Axis 2:\ncontrol mode"=enum."amplitude", "axis 1:\nOutput"=FALSE, "axis 2:\nOutput 2"=FALSE, "axis 1:\nstop detection"=FALSE, "axis 2:\nstop detection"=FALSE, "axis 1:\nSingle Circle Mode"=FALSE, "axis 2:\nSingle Circle Mode"=FALSE, "axis 1: \nTarget GND"=FALSE, "axis 2: \nTarget GND"=FALSE, "Set static Amplitude when moving?"=FALSE, "Static Amplitude (mV)"=0.0} ("Inputs"), "Axes Number"=w341, "Axis 1: Frequency [Hz]"="axis 1:\nFrequency [Hz]") -> (w346:T2)
                n144 = call "To JSON Text.vim"("Anything"=w346) -> ("<JSON>"=w345:string)  [unwired: 9 in, 1 out]
                n145 = Bundle By Name(cluster=w343, "Message.Command"="setFrequency", "Message.Data"=w345) -> (w344:T10)
                n146 = call <vilib>:"Add State(s) to Queue__jki_lib_state_machine.vi"("State(s) in Front (\"\")"="Data: Set UI Cluster\nData: Set Config Cluster\nAction: Send Message to Instrument\nAction: getAll\nUI: Update FP Indicators" ("State(s) in Front (\"\")"), "State(s) in (\"\")"=w351) -> ("States Out"=w350:string)  [unwired: 13 in]
              }
              event "axis 2:\nFrequency [Hz]": Value Change {
                w353 = u8 1 items=["1", "2", "3", "4", "5", "6", "7", "8", "9"] ("axis no")
                n147 = event-data() -> ()  [unwired: 1 in, 6 out]
                n148 = Bundle By Name(cluster=T2 {"Handle"=0, "Axes Number"=0, "Axis 1: sp Position"=0.0, "Axis 2: sp Position"=0.0, "Axis 1: sp rot count"=0, "Axis 2: sp rot count"=0, "Backward or Forward?"=FALSE, "Axis 1: Amplitude [V] "=0.0, "Axis 2: Amplitude [V] "=0.0, "Axis 1: DCLevel [V]"=0.0, "Axis 2: DCLevel [V]"=0.0, "Axis 1: Frequency [Hz]"=0, "Axis 2: Frequency [Hz]"=0, "Axis 1:\ncontrol mode"=enum."amplitude", "Axis 2:\ncontrol mode"=enum."amplitude", "axis 1:\nOutput"=FALSE, "axis 2:\nOutput 2"=FALSE, "axis 1:\nstop detection"=FALSE, "axis 2:\nstop detection"=FALSE, "axis 1:\nSingle Circle Mode"=FALSE, "axis 2:\nSingle Circle Mode"=FALSE, "axis 1: \nTarget GND"=FALSE, "axis 2: \nTarget GND"=FALSE, "Set static Amplitude when moving?"=FALSE, "Static Amplitude (mV)"=0.0} ("Inputs"), "Axes Number"=w353, "Axis 2: Frequency [Hz]"="axis 2:\nFrequency [Hz]") -> (w358:T2)
                n149 = call "To JSON Text.vim"("Anything"=w358) -> ("<JSON>"=w357:string)  [unwired: 9 in, 1 out]
                n150 = Bundle By Name(cluster=w355, "Message.Command"="setFrequency", "Message.Data"=w357) -> (w356:T10)
                n151 = call <vilib>:"Add State(s) to Queue__jki_lib_state_machine.vi"("State(s) in Front (\"\")"="Data: Set UI Cluster\nData: Set Config Cluster\nAction: Send Message to Instrument\nAction: getAll\nUI: Update FP Indicators" ("State(s) in Front (\"\")"), "State(s) in (\"\")"=w363) -> ("States Out"=w362:string)  [unwired: 13 in]
              }
              event "axis 1:\ncap. measure": Value Change {
                w364 = u8 0 items=["1", "2", "3", "4", "5", "6", "7", "8", "9"] ("axis no")
                n152 = event-data() -> ()  [unwired: 1 in, 6 out]
                n153 = Bundle By Name(cluster=T2 {"Handle"=0, "Axes Number"=0, "Axis 1: sp Position"=0.0, "Axis 2: sp Position"=0.0, "Axis 1: sp rot count"=0, "Axis 2: sp rot count"=0, "Backward or Forward?"=FALSE, "Axis 1: Amplitude [V] "=0.0, "Axis 2: Amplitude [V] "=0.0, "Axis 1: DCLevel [V]"=0.0, "Axis 2: DCLevel [V]"=0.0, "Axis 1: Frequency [Hz]"=0, "Axis 2: Frequency [Hz]"=0, "Axis 1:\ncontrol mode"=enum."amplitude", "Axis 2:\ncontrol mode"=enum."amplitude", "axis 1:\nOutput"=FALSE, "axis 2:\nOutput 2"=FALSE, "axis 1:\nstop detection"=FALSE, "axis 2:\nstop detection"=FALSE, "axis 1:\nSingle Circle Mode"=FALSE, "axis 2:\nSingle Circle Mode"=FALSE, "axis 1: \nTarget GND"=FALSE, "axis 2: \nTarget GND"=FALSE, "Set static Amplitude when moving?"=FALSE, "Static Amplitude (mV)"=0.0} ("Inputs"), "Axes Number"=w364) -> (w369:T2)
                n154 = call "To JSON Text.vim"("Anything"=w369) -> ("<JSON>"=w368:string)  [unwired: 9 in, 1 out]
                n155 = Bundle By Name(cluster=w366, "Message.Command"="CapMeasure", "Message.Data"=w368) -> (w367:T10)
                n156 = call <vilib>:"Add State(s) to Queue__jki_lib_state_machine.vi"("State(s) in Front (\"\")"="Data: Set UI Cluster\nData: Set Config Cluster\nAction: Send Message to Instrument\nAction: getAll\nUI: Update FP Indicators" ("State(s) in Front (\"\")"), "State(s) in (\"\")"=w374) -> ("States Out"=w373:string)  [unwired: 13 in]
              }
              event "axis 2:\ncap. measure": Value Change {
                w375 = u8 1 items=["1", "2", "3", "4", "5", "6", "7", "8", "9"] ("axis no")
                n157 = event-data() -> ()  [unwired: 1 in, 6 out]
                n158 = Bundle By Name(cluster=T2 {"Handle"=0, "Axes Number"=0, "Axis 1: sp Position"=0.0, "Axis 2: sp Position"=0.0, "Axis 1: sp rot count"=0, "Axis 2: sp rot count"=0, "Backward or Forward?"=FALSE, "Axis 1: Amplitude [V] "=0.0, "Axis 2: Amplitude [V] "=0.0, "Axis 1: DCLevel [V]"=0.0, "Axis 2: DCLevel [V]"=0.0, "Axis 1: Frequency [Hz]"=0, "Axis 2: Frequency [Hz]"=0, "Axis 1:\ncontrol mode"=enum."amplitude", "Axis 2:\ncontrol mode"=enum."amplitude", "axis 1:\nOutput"=FALSE, "axis 2:\nOutput 2"=FALSE, "axis 1:\nstop detection"=FALSE, "axis 2:\nstop detection"=FALSE, "axis 1:\nSingle Circle Mode"=FALSE, "axis 2:\nSingle Circle Mode"=FALSE, "axis 1: \nTarget GND"=FALSE, "axis 2: \nTarget GND"=FALSE, "Set static Amplitude when moving?"=FALSE, "Static Amplitude (mV)"=0.0} ("Inputs"), "Axes Number"=w375) -> (w380:T2)
                n159 = call "To JSON Text.vim"("Anything"=w380) -> ("<JSON>"=w379:string)  [unwired: 9 in, 1 out]
                n160 = Bundle By Name(cluster=w377, "Message.Command"="CapMeasure", "Message.Data"=w379) -> (w378:T10)
                n161 = call <vilib>:"Add State(s) to Queue__jki_lib_state_machine.vi"("State(s) in Front (\"\")"="Data: Set UI Cluster\nData: Set Config Cluster\nAction: Send Message to Instrument\nAction: getAll\nUI: Update FP Indicators" ("State(s) in Front (\"\")"), "State(s) in (\"\")"=w385) -> ("States Out"=w384:string)  [unwired: 13 in]
              }
              event "axis 1:\ncontrol mode": Value Change {
                w387 = u8 0 items=["1", "2", "3", "4", "5", "6", "7", "8", "9"] ("axis no")
                n162 = event-data() -> ()  [unwired: 1 in, 6 out]
                n163 = Bundle By Name(cluster=T2 {"Handle"=0, "Axes Number"=0, "Axis 1: sp Position"=0.0, "Axis 2: sp Position"=0.0, "Axis 1: sp rot count"=0, "Axis 2: sp rot count"=0, "Backward or Forward?"=FALSE, "Axis 1: Amplitude [V] "=0.0, "Axis 2: Amplitude [V] "=0.0, "Axis 1: DCLevel [V]"=0.0, "Axis 2: DCLevel [V]"=0.0, "Axis 1: Frequency [Hz]"=0, "Axis 2: Frequency [Hz]"=0, "Axis 1:\ncontrol mode"=enum."amplitude", "Axis 2:\ncontrol mode"=enum."amplitude", "axis 1:\nOutput"=FALSE, "axis 2:\nOutput 2"=FALSE, "axis 1:\nstop detection"=FALSE, "axis 2:\nstop detection"=FALSE, "axis 1:\nSingle Circle Mode"=FALSE, "axis 2:\nSingle Circle Mode"=FALSE, "axis 1: \nTarget GND"=FALSE, "axis 2: \nTarget GND"=FALSE, "Set static Amplitude when moving?"=FALSE, "Static Amplitude (mV)"=0.0} ("Inputs"), "Axes Number"=w387, "Axis 1:\ncontrol mode"="axis 1:\ncontrol mode") -> (w392:T2)
                n164 = call "To JSON Text.vim"("Anything"=w392) -> ("<JSON>"=w391:string)  [unwired: 9 in, 1 out]
                n165 = Bundle By Name(cluster=w389, "Message.Command"="AmplitudeControl", "Message.Data"=w391) -> (w390:T10)
                n166 = call <vilib>:"Add State(s) to Queue__jki_lib_state_machine.vi"("State(s) in Front (\"\")"="Data: Set UI Cluster\nData: Set Config Cluster\nAction: Send Message to Instrument\nAction: getAll\nUI: Update FP Indicators" ("State(s) in Front (\"\")"), "State(s) in (\"\")"=w397) -> ("States Out"=w396:string)  [unwired: 13 in]
              }
              event "axis 2:\ncontrol mode": Value Change {
                w399 = u8 1 items=["1", "2", "3", "4", "5", "6", "7", "8", "9"] ("axis no")
                n167 = event-data() -> ()  [unwired: 1 in, 6 out]
                n168 = Bundle By Name(cluster=T2 {"Handle"=0, "Axes Number"=0, "Axis 1: sp Position"=0.0, "Axis 2: sp Position"=0.0, "Axis 1: sp rot count"=0, "Axis 2: sp rot count"=0, "Backward or Forward?"=FALSE, "Axis 1: Amplitude [V] "=0.0, "Axis 2: Amplitude [V] "=0.0, "Axis 1: DCLevel [V]"=0.0, "Axis 2: DCLevel [V]"=0.0, "Axis 1: Frequency [Hz]"=0, "Axis 2: Frequency [Hz]"=0, "Axis 1:\ncontrol mode"=enum."amplitude", "Axis 2:\ncontrol mode"=enum."amplitude", "axis 1:\nOutput"=FALSE, "axis 2:\nOutput 2"=FALSE, "axis 1:\nstop detection"=FALSE, "axis 2:\nstop detection"=FALSE, "axis 1:\nSingle Circle Mode"=FALSE, "axis 2:\nSingle Circle Mode"=FALSE, "axis 1: \nTarget GND"=FALSE, "axis 2: \nTarget GND"=FALSE, "Set static Amplitude when moving?"=FALSE, "Static Amplitude (mV)"=0.0} ("Inputs"), "Axes Number"=w399, "Axis 1:\ncontrol mode"="axis 2:\ncontrol mode") -> (w404:T2)
                n169 = call "To JSON Text.vim"("Anything"=w404) -> ("<JSON>"=w403:string)  [unwired: 9 in, 1 out]
                n170 = Bundle By Name(cluster=w401, "Message.Command"="AmplitudeControl", "Message.Data"=w403) -> (w402:T10)
                n171 = call <vilib>:"Add State(s) to Queue__jki_lib_state_machine.vi"("State(s) in Front (\"\")"="Data: Set UI Cluster\nData: Set Config Cluster\nAction: Send Message to Instrument\nAction: getAll\nUI: Update FP Indicators" ("State(s) in Front (\"\")"), "State(s) in (\"\")"=w409) -> ("States Out"=w408:string)  [unwired: 13 in]
              }
              event "axis 1:\nOutput": Value Change {
                w411 = u8 0 items=["1", "2", "3", "4", "5", "6", "7", "8", "9"] ("axis no")
                n172 = event-data() -> ()  [unwired: 1 in, 6 out]
                n173 = Bundle By Name(cluster=T2 {"Handle"=0, "Axes Number"=0, "Axis 1: sp Position"=0.0, "Axis 2: sp Position"=0.0, "Axis 1: sp rot count"=0, "Axis 2: sp rot count"=0, "Backward or Forward?"=FALSE, "Axis 1: Amplitude [V] "=0.0, "Axis 2: Amplitude [V] "=0.0, "Axis 1: DCLevel [V]"=0.0, "Axis 2: DCLevel [V]"=0.0, "Axis 1: Frequency [Hz]"=0, "Axis 2: Frequency [Hz]"=0, "Axis 1:\ncontrol mode"=enum."amplitude", "Axis 2:\ncontrol mode"=enum."amplitude", "axis 1:\nOutput"=FALSE, "axis 2:\nOutput 2"=FALSE, "axis 1:\nstop detection"=FALSE, "axis 2:\nstop detection"=FALSE, "axis 1:\nSingle Circle Mode"=FALSE, "axis 2:\nSingle Circle Mode"=FALSE, "axis 1: \nTarget GND"=FALSE, "axis 2: \nTarget GND"=FALSE, "Set static Amplitude when moving?"=FALSE, "Static Amplitude (mV)"=0.0} ("Inputs"), "Axes Number"=w411, "axis 1:\nOutput"="axis 1:\nOutput") -> (w416:T2)
                n174 = call "To JSON Text.vim"("Anything"=w416) -> ("<JSON>"=w415:string)  [unwired: 9 in, 1 out]
                n175 = Bundle By Name(cluster=w413, "Message.Command"="SetOutput", "Message.Data"=w415) -> (w414:T10)
                n176 = call <vilib>:"Add State(s) to Queue__jki_lib_state_machine.vi"("State(s) in Front (\"\")"="Data: Set UI Cluster\nData: Set Config Cluster\nAction: Send Message to Instrument\nAction: getAll\nUI: Update FP Indicators" ("State(s) in Front (\"\")"), "State(s) in (\"\")"=w421) -> ("States Out"=w420:string)  [unwired: 13 in]
              }
              event "axis 2:\nOutput": Value Change {
                w423 = u8 1 items=["1", "2", "3", "4", "5", "6", "7", "8", "9"] ("axis no")
                n177 = event-data() -> ()  [unwired: 1 in, 6 out]
                n178 = Bundle By Name(cluster=T2 {"Handle"=0, "Axes Number"=0, "Axis 1: sp Position"=0.0, "Axis 2: sp Position"=0.0, "Axis 1: sp rot count"=0, "Axis 2: sp rot count"=0, "Backward or Forward?"=FALSE, "Axis 1: Amplitude [V] "=0.0, "Axis 2: Amplitude [V] "=0.0, "Axis 1: DCLevel [V]"=0.0, "Axis 2: DCLevel [V]"=0.0, "Axis 1: Frequency [Hz]"=0, "Axis 2: Frequency [Hz]"=0, "Axis 1:\ncontrol mode"=enum."amplitude", "Axis 2:\ncontrol mode"=enum."amplitude", "axis 1:\nOutput"=FALSE, "axis 2:\nOutput 2"=FALSE, "axis 1:\nstop detection"=FALSE, "axis 2:\nstop detection"=FALSE, "axis 1:\nSingle Circle Mode"=FALSE, "axis 2:\nSingle Circle Mode"=FALSE, "axis 1: \nTarget GND"=FALSE, "axis 2: \nTarget GND"=FALSE, "Set static Amplitude when moving?"=FALSE, "Static Amplitude (mV)"=0.0} ("Inputs"), "Axes Number"=w423, "axis 1:\nOutput"="axis 2:\nOutput") -> (w428:T2)
                n179 = call "To JSON Text.vim"("Anything"=w428) -> ("<JSON>"=w427:string)  [unwired: 9 in, 1 out]
                n180 = Bundle By Name(cluster=w425, "Message.Command"="SetOutput", "Message.Data"=w427) -> (w426:T10)
                n181 = call <vilib>:"Add State(s) to Queue__jki_lib_state_machine.vi"("State(s) in Front (\"\")"="Data: Set UI Cluster\nData: Set Config Cluster\nAction: Send Message to Instrument\nAction: getAll\nUI: Update FP Indicators" ("State(s) in Front (\"\")"), "State(s) in (\"\")"=w433) -> ("States Out"=w432:string)  [unwired: 13 in]
              }
              event "axis 1:\nstop detection": Value Change {
                w435 = u8 0 items=["1", "2", "3", "4", "5", "6", "7", "8", "9"] ("axis no")
                n182 = event-data() -> ()  [unwired: 1 in, 6 out]
                n183 = Bundle By Name(cluster=T2 {"Handle"=0, "Axes Number"=0, "Axis 1: sp Position"=0.0, "Axis 2: sp Position"=0.0, "Axis 1: sp rot count"=0, "Axis 2: sp rot count"=0, "Backward or Forward?"=FALSE, "Axis 1: Amplitude [V] "=0.0, "Axis 2: Amplitude [V] "=0.0, "Axis 1: DCLevel [V]"=0.0, "Axis 2: DCLevel [V]"=0.0, "Axis 1: Frequency [Hz]"=0, "Axis 2: Frequency [Hz]"=0, "Axis 1:\ncontrol mode"=enum."amplitude", "Axis 2:\ncontrol mode"=enum."amplitude", "axis 1:\nOutput"=FALSE, "axis 2:\nOutput 2"=FALSE, "axis 1:\nstop detection"=FALSE, "axis 2:\nstop detection"=FALSE, "axis 1:\nSingle Circle Mode"=FALSE, "axis 2:\nSingle Circle Mode"=FALSE, "axis 1: \nTarget GND"=FALSE, "axis 2: \nTarget GND"=FALSE, "Set static Amplitude when moving?"=FALSE, "Static Amplitude (mV)"=0.0} ("Inputs"), "Axes Number"=w435, "axis 1:\nstop detection"="axis 1:\nstop detection") -> (w440:T2)
                n184 = call "To JSON Text.vim"("Anything"=w440) -> ("<JSON>"=w439:string)  [unwired: 9 in, 1 out]
                n185 = Bundle By Name(cluster=w437, "Message.Command"="StopDetection", "Message.Data"=w439) -> (w438:T10)
                n186 = call <vilib>:"Add State(s) to Queue__jki_lib_state_machine.vi"("State(s) in Front (\"\")"="Data: Set UI Cluster\nData: Set Config Cluster\nAction: Send Message to Instrument\nAction: getAll\nUI: Update FP Indicators" ("State(s) in Front (\"\")"), "State(s) in (\"\")"=w445) -> ("States Out"=w444:string)  [unwired: 13 in]
              }
              event "axis 2:\nstop detection": Value Change {
                w447 = u8 1 items=["1", "2", "3", "4", "5", "6", "7", "8", "9"] ("axis no")
                n187 = event-data() -> ()  [unwired: 1 in, 6 out]
                n188 = Bundle By Name(cluster=T2 {"Handle"=0, "Axes Number"=0, "Axis 1: sp Position"=0.0, "Axis 2: sp Position"=0.0, "Axis 1: sp rot count"=0, "Axis 2: sp rot count"=0, "Backward or Forward?"=FALSE, "Axis 1: Amplitude [V] "=0.0, "Axis 2: Amplitude [V] "=0.0, "Axis 1: DCLevel [V]"=0.0, "Axis 2: DCLevel [V]"=0.0, "Axis 1: Frequency [Hz]"=0, "Axis 2: Frequency [Hz]"=0, "Axis 1:\ncontrol mode"=enum."amplitude", "Axis 2:\ncontrol mode"=enum."amplitude", "axis 1:\nOutput"=FALSE, "axis 2:\nOutput 2"=FALSE, "axis 1:\nstop detection"=FALSE, "axis 2:\nstop detection"=FALSE, "axis 1:\nSingle Circle Mode"=FALSE, "axis 2:\nSingle Circle Mode"=FALSE, "axis 1: \nTarget GND"=FALSE, "axis 2: \nTarget GND"=FALSE, "Set static Amplitude when moving?"=FALSE, "Static Amplitude (mV)"=0.0} ("Inputs"), "Axes Number"=w447, "axis 1:\nstop detection"="axis 2:\nstop detection") -> (w452:T2)
                n189 = call "To JSON Text.vim"("Anything"=w452) -> ("<JSON>"=w451:string)  [unwired: 9 in, 1 out]
                n190 = Bundle By Name(cluster=w449, "Message.Command"="StopDetection", "Message.Data"=w451) -> (w450:T10)
                n191 = call <vilib>:"Add State(s) to Queue__jki_lib_state_machine.vi"("State(s) in Front (\"\")"="Data: Set UI Cluster\nData: Set Config Cluster\nAction: Send Message to Instrument\nAction: getAll\nUI: Update FP Indicators" ("State(s) in Front (\"\")"), "State(s) in (\"\")"=w457) -> ("States Out"=w456:string)  [unwired: 13 in]
              }
              event "axis 1:\nStop moving": Value Change {
                w458 = u8 0 items=["1", "2", "3", "4", "5", "6", "7", "8", "9"] ("axis no")
                n192 = event-data() -> ()  [unwired: 1 in, 6 out]
                n193 = Bundle By Name(cluster=T2 {"Handle"=0, "Axes Number"=0, "Axis 1: sp Position"=0.0, "Axis 2: sp Position"=0.0, "Axis 1: sp rot count"=0, "Axis 2: sp rot count"=0, "Backward or Forward?"=FALSE, "Axis 1: Amplitude [V] "=0.0, "Axis 2: Amplitude [V] "=0.0, "Axis 1: DCLevel [V]"=0.0, "Axis 2: DCLevel [V]"=0.0, "Axis 1: Frequency [Hz]"=0, "Axis 2: Frequency [Hz]"=0, "Axis 1:\ncontrol mode"=enum."amplitude", "Axis 2:\ncontrol mode"=enum."amplitude", "axis 1:\nOutput"=FALSE, "axis 2:\nOutput 2"=FALSE, "axis 1:\nstop detection"=FALSE, "axis 2:\nstop detection"=FALSE, "axis 1:\nSingle Circle Mode"=FALSE, "axis 2:\nSingle Circle Mode"=FALSE, "axis 1: \nTarget GND"=FALSE, "axis 2: \nTarget GND"=FALSE, "Set static Amplitude when moving?"=FALSE, "Static Amplitude (mV)"=0.0} ("Inputs"), "Axes Number"=w458) -> (w463:T2)
                n194 = call "To JSON Text.vim"("Anything"=w463) -> ("<JSON>"=w462:string)  [unwired: 9 in, 1 out]
                n195 = Bundle By Name(cluster=w460, "Message.Command"="StopMoving", "Message.Data"=w462) -> (w461:T10)
                n196 = call <vilib>:"Add State(s) to Queue__jki_lib_state_machine.vi"("State(s) in Front (\"\")"="Data: Set UI Cluster\nData: Set Config Cluster\nAction: Send Message to Instrument\nAction: getAll\nUI: Update FP Indicators" ("State(s) in Front (\"\")"), "State(s) in (\"\")"=w468) -> ("States Out"=w467:string)  [unwired: 13 in]
              }
              event "axis 2:\nStop moving": Value Change {
                w469 = u8 1 items=["1", "2", "3", "4", "5", "6", "7", "8", "9"] ("axis no")
                n197 = event-data() -> ()  [unwired: 1 in, 6 out]
                n198 = Bundle By Name(cluster=T2 {"Handle"=0, "Axes Number"=0, "Axis 1: sp Position"=0.0, "Axis 2: sp Position"=0.0, "Axis 1: sp rot count"=0, "Axis 2: sp rot count"=0, "Backward or Forward?"=FALSE, "Axis 1: Amplitude [V] "=0.0, "Axis 2: Amplitude [V] "=0.0, "Axis 1: DCLevel [V]"=0.0, "Axis 2: DCLevel [V]"=0.0, "Axis 1: Frequency [Hz]"=0, "Axis 2: Frequency [Hz]"=0, "Axis 1:\ncontrol mode"=enum."amplitude", "Axis 2:\ncontrol mode"=enum."amplitude", "axis 1:\nOutput"=FALSE, "axis 2:\nOutput 2"=FALSE, "axis 1:\nstop detection"=FALSE, "axis 2:\nstop detection"=FALSE, "axis 1:\nSingle Circle Mode"=FALSE, "axis 2:\nSingle Circle Mode"=FALSE, "axis 1: \nTarget GND"=FALSE, "axis 2: \nTarget GND"=FALSE, "Set static Amplitude when moving?"=FALSE, "Static Amplitude (mV)"=0.0} ("Inputs"), "Axes Number"=w469) -> (w474:T2)
                n199 = call "To JSON Text.vim"("Anything"=w474) -> ("<JSON>"=w473:string)  [unwired: 9 in, 1 out]
                n200 = Bundle By Name(cluster=w471, "Message.Command"="StopMoving", "Message.Data"=w473) -> (w472:T10)
                n201 = call <vilib>:"Add State(s) to Queue__jki_lib_state_machine.vi"("State(s) in Front (\"\")"="Data: Set UI Cluster\nData: Set Config Cluster\nAction: Send Message to Instrument\nAction: getAll\nUI: Update FP Indicators" ("State(s) in Front (\"\")"), "State(s) in (\"\")"=w479) -> ("States Out"=w478:string)  [unwired: 13 in]
              }
              event "static amplitude (mV)": Value Change {
                n202 = event-data() -> ()  [unwired: 1 in, 6 out]
                n203 = local read "set static amplitude\nwhen moving"() -> (w480:bool)
                n204 = Bundle By Name(cluster=T2 {"Handle"=0, "Axes Number"=0, "Axis 1: sp Position"=0.0, "Axis 2: sp Position"=0.0, "Axis 1: sp rot count"=0, "Axis 2: sp rot count"=0, "Backward or Forward?"=FALSE, "Axis 1: Amplitude [V] "=0.0, "Axis 2: Amplitude [V] "=0.0, "Axis 1: DCLevel [V]"=0.0, "Axis 2: DCLevel [V]"=0.0, "Axis 1: Frequency [Hz]"=0, "Axis 2: Frequency [Hz]"=0, "Axis 1:\ncontrol mode"=enum."amplitude", "Axis 2:\ncontrol mode"=enum."amplitude", "axis 1:\nOutput"=FALSE, "axis 2:\nOutput 2"=FALSE, "axis 1:\nstop detection"=FALSE, "axis 2:\nstop detection"=FALSE, "axis 1:\nSingle Circle Mode"=FALSE, "axis 2:\nSingle Circle Mode"=FALSE, "axis 1: \nTarget GND"=FALSE, "axis 2: \nTarget GND"=FALSE, "Set static Amplitude when moving?"=FALSE, "Static Amplitude (mV)"=0.0} ("Inputs"), "Set static Amplitude when moving?"=w480, "Static Amplitude (mV)"="static amplitude (mV)") -> (w486:T2)
                n205 = call "To JSON Text.vim"("Anything"=w486) -> ("<JSON>"=w485:string)  [unwired: 9 in, 1 out]
                n206 = Bundle By Name(cluster=w483, "Message.Command"="StaticAmplitude", "Message.Data"=w485) -> (w484:T10)
                n207 = call <vilib>:"Add State(s) to Queue__jki_lib_state_machine.vi"("State(s) in Front (\"\")"="Data: Set UI Cluster\nData: Set Config Cluster\nAction: Send Message to Instrument\nAction: getAll\nUI: Update FP Indicators" ("State(s) in Front (\"\")"), "State(s) in (\"\")"=w491) -> ("States Out"=w490:string)  [unwired: 13 in]
              }
              event User Event {
                # "Handle messages from Instrument:process.vi"
                n208 = event-data() -> ("Message"=w492:T9)  [unwired: 1 in, 4 out]
                n209 = Bundle By Name(cluster=w495, "Message"=w492) -> (w494:T10)
                n210 = call <vilib>:"Add State(s) to Queue__jki_lib_state_machine.vi"("State(s) in Front (\"\")"="" ("State(s) in Front (\"\")"), "State(s) in (\"\")"=w498) -> ("States Out"=w497:string)  [unwired: 13 in]
              }
              event User Event {
                # "Handle messages from Inst.child:process.vi"
                n211 = event-data() -> ("Message"=w499:T9)  [unwired: 1 in, 4 out]
                n212 = Bundle By Name(cluster=w502, "Message"=w499) -> (w501:T10)
                n213 = call <vilib>:"Add State(s) to Queue__jki_lib_state_machine.vi"("State(s) in Front (\"\")"="" ("State(s) in Front (\"\")"), "State(s) in (\"\")"=w505) -> ("States Out"=w504:string)  [unwired: 13 in]
              }
              event Panel Close? {
                # "Discard the event because we'll close the front panel ourselves in Macro: Exit"
                # "Close Panel button (pressed) Event\n(this executes Macro: Exit to terminate the VI)"
                n214 = event-data() -> ()  [unwired: 1 in, 1 out]
                n215 = event-data("Discard?"=FALSE) -> ()  [unwired: 1 in, 1 out]
                n216 = call <vilib>:"Add State(s) to Queue__jki_lib_state_machine.vi"("State(s) in Front (\"\")"="Action: Notify UI Closed\nMacro: Exit", "State(s) in (\"\")"=w511) -> ("States Out"=w510:string)  [unwired: 13 in]
              }
              event User Event {
                n217 = event-data() -> ()  [unwired: 1 in, 5 out]
                n218 = call <vilib>:"Add State(s) to Queue__jki_lib_state_machine.vi"("State(s) in Front (\"\")"="Macro: Exit", "State(s) in (\"\")"=w516) -> ("States Out"=w515:string)  [unwired: 13 in]
              }
              event User Event {
                # "On Abort, no nice macro exit, but exit right away"
                n219 = event-data() -> ()  [unwired: 1 in, 5 out]
                n220 = call <vilib>:"Add State(s) to Queue__jki_lib_state_machine.vi"("State(s) in Front (\"\")"="Exit", "State(s) in (\"\")"=w521) -> ("States Out"=w520:string)  [unwired: 13 in]
              }
              event "Exit": Value Change {
                # "On Abort, no nice macro exit, but exit right away"
                n221 = event-data() -> ()  [unwired: 1 in, 6 out]
                n222 = Two Button Dialog(message="Are you sure you want to stop this program?") -> (T button?=w526:bool)  [unwired: 2 in]
                n223 = Select(t="Macro: Exit", s=w526, f="") -> (s? t:f=w522:string)
                n224 = call <vilib>:"Add State(s) to Queue__jki_lib_state_machine.vi"("State(s) in Front (\"\")"=w522, "State(s) in (\"\")"=w530) -> ("States Out"=w529:string)  [unwired: 13 in]
              }
            }
          }
          frame "---------- Core ----------" {
            # "Do not put any code in this frame.\n(it is a separator no-op)"
            n225 = call <vilib>:"Add State(s) to Queue__jki_lib_state_machine.vi"("State(s) in (\"\")"=w535) -> ("States Out"=w534:string)  [unwired: 14 in]
          }
          frame Default {
            w546 = 42 items=["No error", "Argument error", "Memory is full", "Out of zone", "End of file", "File already open", "Generic file I/O error", "File not found", "File permission error", "Disk is full", "Duplicate path", "Too many files open", "System feature not enabled", "Resource file not found", "Cannot add resource", "Resource not found", "Image not found", "Image memory error", "Pen does not exist", "Config type invalid", "Config token not found", "Config parse error", "Config memory error", "Bad external code format", "Bad external code offset", "External code not present", "Null window", "Destroy window error", "Null menu", "Print aborted", "Bad print record", "Print driver error", "Windows error during printing", "Memory error during printing", "Print dialog error", "Generic print error", "Invalid device refnum", "Device not found", "Device parameter error", "Device unit error", "Cannot open device", "Device call aborted", "Generic error", "Cancelled by user", "Object ID too low", "Object ID too high", "Object not in heap", "Unknown heap", "Unknown object (invalid DefProc)", "Unknown object (DefProc not in table)", "Message out of range", "Invalid (null) method", "Unknown message", "Manager call not supported", "Bad address", "Network operation in progress", "Network operation timed out", "Connection is busy", "Network attribute not supported", "Network error", "Address in use", "System out of memory", "Connection aborted", "Connection refused", "Not connected", "Already connected", "Connection closed", "Initialization error (interapplication manager)", "Bad occurrence", "Wait on unbound occurrence handler", "Occurrence queue overflow", "Datalog type conflict", "Unused", "Unrecognized type (interapplication manager)", "Memory corrupt", "Failed to make temporary DLL", "Old CIN version", "Drag socket not found", "Failed to load drop-object", "Failed to register OLE object", "Failed to release OLE object", "Format specifier type mismatch", "Unknown format specifier", "Too few format specifiers", "Too many format specifiers", "Scan failed", "Newer CIN version", "Error converting to variant", "Runtime menu error", "Password tampered", "Variant attribute not found", "Incompatible variant data type", "Event data is not available", "Event Store is not present", "Occurrence is not found", "Event Queue is not created", "Event info is not available", "Refnum passed is NULL", "Error retrieving Class GUID", "Error retrieving CoClass GUID", "Error retrieving TypeLib GUID.", "Bad built application magic bytes.", "Specific driver is different from the specific driver associated with the Logical Name.", "There is no session opened to the class driver.", "Max Error", "MAX - Error with config objects", "MAX - Error loading configuration", "MAX - Group not supported"]
            # "Current State"
            # "Do not delete, rename, or modify this frame.\n(this is used to capture unhandled states and typos)"
            # "Handle mistyped state name (developer tool)"
            n226 = Format Into String(format string="Software Exception: Unhandled State \"%s\"." ("message"), error in=w542, w537) -> (resulting string=w545:string, error out=w544:errorcluster)  [unwired: 1 in]
            n227 = call <vilib>:"Error Cluster From Error Code.vi"("show call chain? (False)"=TRUE, "error in (no error)"=w544, "error message (\"\")"=w545, "error code (0)"=w546) -> ("error out"=w543:errorcluster)  [unwired: 5 in]
            n228 = call <vilib>:"Add State(s) to Queue__jki_lib_state_machine.vi"("State(s) in (\"\")"=w541) -> ("States Out"=w540:string)  [unwired: 14 in]
          }
          frame "Initialize Core Data" {
            # "Do not delete, rename, or modify this frame.\n(this is used to determine panel behavior on exit)"
            # "originally closed?"
            # "exe?"
            # "If panel starts closed or is an EXE, then close it when we exit"
            n229 = property class="VI"() -> ("Front Panel.Open"=w556:bool)  [unwired: 2 in, 2 out]
            n230 = property class="App"() -> ("App.Kind"=w555:T3)  [unwired: 2 in, 2 out]
            n231 = control-ref of="Current VI Reference"() -> (w549:refnum<vi>)
            n232 = Not(x=w556) -> (.not. x?=w553:bool)
            n233 = Equal?(x=w555, y=T3."Run Time System" ("Application:Kind")) -> (x = y?=w552:bool)
            n234 = Or(x=w553, y=w552) -> (x .or. y?=w550:bool)
            n235 = Bundle By Name(cluster=w551, "Core.Current VI Reference"=w549, "Core.Close Panel on Exit?"=w550) -> (w558:T10)
            n236 = call <vilib>:"Add State(s) to Queue__jki_lib_state_machine.vi"("State(s) in (\"\")"=w560) -> ("States Out"=w559:string)  [unwired: 14 in]
          }
          frame "Error Handler" {
            w569 = errorcluster {"status"=FALSE, "code"=0, "source"=""}  # No error
            # "Overwrite this method to handle errors and pass to parent if not handled. Parent will fire a public event if the error is not handled up the chain of classes."
            # "Handle any errors here.\nYou can also output any states to clean-up after errors occur"
            n237 = Unbundle By Name(w567) -> ("Instrument UI"=w572:refnum<class "Inst UI.Attocube-3DR.lvclass">)
            n238 = call-dynamic "Handle Error.vi"("Stop on Unhandled Error (T)"=FALSE, "error in"=w563, "SMO"=w572) -> ("handling error"=w570:errorcluster, "Unhandled error"=w568:errorcluster)  [unwired: 6 in, 1 out]
            n239 = Bundle By Name(cluster=w567, "Core.Last Error.remaining states"=w564, "Core.Last Error.error"=w568) -> (w566:T10)
            n240 = Select(t="Exit", s=w570, f="Macro: Post Error Handling") -> (s? t:f=w561:string)
          }
          frame "Exit" {
            # "Do not put any code in this frame.\n(No errors that occur here will be handled.)"
            n241 = Unbundle By Name(w575) -> ("Core.Last Error.error"=w574:errorcluster)
            n242 = call <vilib>:"Add State(s) to Queue__jki_lib_state_machine.vi"("State(s) in (\"\")"=w579) -> ("States Out"=w578:string)  [unwired: 14 in]
          }
          frame "---------- Data ----------" {
            # "Do not put any code in this frame.\n(It is a separator no-op. You can make a copy of this frame to create a new Data frame)"
            n243 = call <vilib>:"Add State(s) to Queue__jki_lib_state_machine.vi"("State(s) in (\"\")"=w584) -> ("States Out"=w583:string)  [unwired: 14 in]
          }
          frame "Data: Initialize" {
            w585 = T9 {"Command"="", "Data"=variant, "ID"=""}  # Message
            w588 = refnum<class "Configuration.lvclass"> refnum  # Configuration
            w591 = T6 {"Example Setting 1"=0.0, "Example Setting 2"=0.0, "Example Setting 3"=""}  # Config Cluster
            w593 = T8 {"static amplitude (mV)"=0.0, "Axis1"={"axis 1:\nsp rot count"=0, "axis 1:\nsp position °"=167.0, "axis 1:\nAmplitude [V]"=40.0, "axis 1:\nDCLevel [V]"=0.0, "axis 1:\nFrequency [Hz]"=800}, "Axis2"={"axis 2:\nsp rot count"=0, "axis2:\nsp position °"=167.0, "axis 2:\nAmplitude [V]"=40.0, "axis 2:\nDCLevel [V]"=0.0, "axis 2:\nFrequency [Hz]"=800}}  # UI Cluster
            w595 = refnum<class "Inst.Attocube-3DR.lvclass"> refnum  # Instrument
            w597 = T7 {"Axis 1: Amplitude"=0, "Axis 1: Capacitance"=0, "Axis 1: Current Position"=0, "Axis 1: DCLevel"=0, "Axis 1: Frequency"=0, "Axis 1: StepWidth"=0, "Axis 1: control mode"=0, "Axis 1: rot. count"=0, "Axis 1: sp position"=0, "Axis 1: sp rot. count"=0, "Axis 1: speed"=0, "Axis 1: Target GND"=FALSE, "Axis 1: Output"=FALSE, "Axis 1: Single Circle Mode"=FALSE, "Axis 1: moving"=FALSE, "Axis 1: stop detected"=FALSE, "Axis 1:  sensor error"=FALSE, "Axis 1: sensor diconnected"=FALSE, "Axis 1: stop enable"=FALSE, "Axis 2: Current Position"=0, "Axis 2: DCLevel"=0, "Axis 2: Frequency"=0, "Axis 2: StepWidth"=0, "Axis 2: control mode"=0, "Axis 2: rot. count"=0, "Axis 2: sp position"=0, "Axis 2: sp rot. count"=0, "Axis 2: speed"=0, "Axis 2: Capacitance"=0, "Axis 2: Amplitude"=0, "Axis 2: Target GND"=FALSE, "Axis 2: Output"=FALSE, "Axis 2: Single Circle Mode"=FALSE, "Axis 2: moving"=FALSE, "Axis 2: stop detected"=FALSE, "Axis 2:  sensor error"=FALSE, "Axis 2: sensor diconnected"=FALSE, "Axis 2: stop enable"=FALSE}  # getAll
            w598 = T11 {"Current VI Reference"=refnum, "Close Panel on Exit?"=FALSE, "Last Error"={"error"={"status"=FALSE, "code"=0, "source"=""}, "previous state"="", "remaining states"=""}, "Shutdown?"=FALSE}  # Core
            # "typedef from Child Instrument"
            # "Cluster of UI\ninformation you\nwant to save/load"
            # "Child Instrument"
            # "typedef from Child Instrument"
            # "do not delete - used by framework"
            # "Data names and types of shift register data are defined by this bundle."
            # "Initialize the shift-register data, here.\n(data names are defined by what you wire into the bundle function)"
            n244 = call <userlib>:"Read Instrument.vi"("error in (no error)"=w586, "Instrument UI in"=w587) -> ("error out"=w592:errorcluster, "Instrument"=w594:refnum<class "Instrument.lvclass">, "Instrument UI"=w596:refnum<class "Inst UI.Attocube-3DR.lvclass">)  [unwired: 7 in]
            n245 = To More Specific Class(target class=w595, reference=w594, error in=w592) -> (specific class reference=w590:refnum<class "Inst.Attocube-3DR.lvclass">, error out=w589:errorcluster)
            n246 = Bundle("Core"=w598, "Instrument UI"=w596, "Instrument"=w590, "Configuration"=w588, "Config Cluster"=w591, "getAll"=w597, "UI Cluster"=w593, "Message"=w585) -> (w600:T10)  [unwired: 1 in]
            n247 = call <vilib>:"Add State(s) to Queue__jki_lib_state_machine.vi"("State(s) in (\"\")"=w602) -> ("States Out"=w601:string)  [unwired: 14 in]
          }
          frame "Data: Set UI Cluster" {
            # "Do not put any code in this frame.\n(It is a separator no-op. You can make a copy of this frame to create a new Data frame)"
            n248 = local read "axis 2:\nFrequency [Hz]"() -> (w603:i32)
            n249 = local read "axis 2:\nAmplitude [V]"() -> (w605:dbl)
            n250 = local read "axis 2:\nsp rot count"() -> (w607:dbl)
            n251 = local read "axis 2:\nsp position °"() -> (w606:i32)
            n252 = local read "axis 2:\nDCLevel [V]"() -> (w604:dbl)
            n253 = Bundle By Name(cluster=w613, "UI Cluster.Axis2.axis 2:\nsp rot count"=w607, "UI Cluster.Axis2.axis2:\nsp position °"=w606, "UI Cluster.Axis2.axis 2:\nAmplitude [V]"=w605, "UI Cluster.Axis2.axis 2:\nDCLevel [V]"=w604, "UI Cluster.Axis2.axis 2:\nFrequency [Hz]"=w603) -> (w614:T10)
            n254 = local read "axis 1:\nsp position °"() -> (w610:dbl)
            n255 = local read "axis 1:\nsp rot count"() -> (w609:i32)
            n256 = local read "axis 1:\nFrequency [Hz]"() -> (w608:i32)
            n257 = local read "axis 1:\nAmplitude [V]"() -> (w611:dbl)
            n258 = local read "axis 1:\nDCLevel [V]"() -> (w612:dbl)
            n259 = Bundle By Name(cluster=w614, "UI Cluster.Axis1.axis 1:\nsp rot count"=w609, "UI Cluster.Axis1.axis 1:\nsp position °"=w610, "UI Cluster.Axis1.axis 1:\nAmplitude [V]"=w611, "UI Cluster.Axis1.axis 1:\nDCLevel [V]"=w612, "UI Cluster.Axis1.axis 1:\nFrequency [Hz]"=w608) -> (w615:T10)
            n260 = call <vilib>:"Add State(s) to Queue__jki_lib_state_machine.vi"("State(s) in (\"\")"=w619) -> ("States Out"=w618:string)  [unwired: 14 in]
          }
          frame "Data: Set Config Cluster" {
            # "Do not put any code in this frame.\n(It is a separator no-op. You can make a copy of this frame to create a new Data frame)"
            n261 = Unbundle By Name(w623) -> ("UI Cluster.Axis1.axis 1:\nsp rot count"=w621:i32)
            n262 = Square(x=w621) -> (x^2=w620:i32)
            n263 = Bundle By Name(cluster=w623, "Config Cluster.Example Setting 1"=w621, "Config Cluster.Example Setting 2"=w620) -> (w622:T10)
            n264 = call <vilib>:"Add State(s) to Queue__jki_lib_state_machine.vi"("State(s) in (\"\")"=w627) -> ("States Out"=w626:string)  [unwired: 14 in]
          }
          frame "Data: Cleanup" {
            # "Cleanup any data and references, here.\n(this is called automatically, by the Macro: Exit)"
            n265 = Unbundle By Name(w628) -> ("Core.Current VI Reference"=w632:refnum<vi>)
            n266 = Close Reference(reference=w632, error in (no error)=w631) -> (error out=w630:errorcluster)
            n267 = call <vilib>:"Add State(s) to Queue__jki_lib_state_machine.vi"("State(s) in (\"\")"=w634) -> ("States Out"=w633:string)  [unwired: 14 in]
          }
          frame "---------- UI ----------" {
            # "Do not put any code in this frame.\n(It is a separator no-op. You can make a copy of this frame to create a new UI frame)"
            n268 = call <vilib>:"Add State(s) to Queue__jki_lib_state_machine.vi"("State(s) in (\"\")"=w639) -> ("States Out"=w638:string)  [unwired: 14 in]
          }
          frame "UI: Initialize" {
            # "size window to decoration box on front panel"
            # "Initialize the User Interface, here.\n(this is called automatically, by the Macro: Init)"
            n269 = call <userlib>:"Fit VI window to Largest Dec__ogtk.vi"("error in (no error)"=w642, "border spacing (2 px)"=0) -> ("error out"=w641:errorcluster)  [unwired: 4 in, 1 out]
            n270 = call <vilib>:"Add State(s) to Queue__jki_lib_state_machine.vi"("State(s) in (\"\")"=w646) -> ("States Out"=w645:string)  [unwired: 14 in]
          }
          frame "UI: Update FP Controls" {
            # "Do not put any code in this frame.\n(It is a separator no-op. You can make a copy of this frame to create a new UI frame)"
            n271 = Unbundle By Name(w655) -> ("UI Cluster.Axis1.axis 1:\nsp rot count"=w657:i32, "UI Cluster.Axis1.axis 1:\nsp position °"=w656:dbl, "UI Cluster.Axis1.axis 1:\nAmplitude [V]"=w654:dbl, "UI Cluster.Axis1.axis 1:\nDCLevel [V]"=w653:dbl, "UI Cluster.Axis1.axis 1:\nFrequency [Hz]"=w652:i32)
            n272 = Unbundle By Name(w655) -> ("UI Cluster.static amplitude (mV)"=w658:dbl)
            n273 = Unbundle By Name(w655) -> ("UI Cluster.Axis2.axis 2:\nsp rot count"=w648:i32, "UI Cluster.Axis2.axis2:\nsp position °"=w651:dbl, "UI Cluster.Axis2.axis 2:\nAmplitude [V]"=w647:dbl, "UI Cluster.Axis2.axis 2:\nDCLevel [V]"=w649:dbl, "UI Cluster.Axis2.axis 2:\nFrequency [Hz]"=w650:i32)
            n274 = local write "axis 1:\nsp rot count"(w657) -> ()
            n275 = local write "axis 1:\nsp position °"(w656) -> ()
            n276 = local write "static amplitude (mV)"(w658) -> ()
            n277 = local write "axis 2:\nAmplitude [V]"(w654) -> ()
            n278 = local write "axis 1:\nDCLevel [V]"(w653) -> ()
            n279 = local write "axis 1:\nFrequency [Hz]"(w652) -> ()
            n280 = local write "axis 2:\nAmplitude [V]"(w647) -> ()
            n281 = local write "axis 2:\nDCLevel [V]"(w649) -> ()
            n282 = local write "axis 2:\nFrequency [Hz]"(w650) -> ()
            n283 = local write "axis 2:\nsp rot count"(w648) -> ()
            n284 = local write "axis 2:\nsp position °"(w651) -> ()
            n285 = call <vilib>:"Add State(s) to Queue__jki_lib_state_machine.vi"("State(s) in (\"\")"=w662) -> ("States Out"=w661:string)  [unwired: 14 in]
          }
          frame "UI: Update FP Indicators" {
            # "current position indicators to be editted later"
            # "do this way to have nicer UI or only display what you want"
            n286 = Unbundle By Name(w691) -> ("getAll"=w693:T7)
            n287 = Unbundle By Name(w693) -> ("Axis 1: Capacitance"=→"Axis 1: Capacitance [nF]":i32, "Axis 1: rot. count"=→"Axis 1: rot. count":i32, "Axis 1: Current Position"=→"axis 1:\nCurrent position [µm/°/m°] 2" →"Axis 1: Current Position (°)":i32, "Axis 1: StepWidth"=→"Axis 1: StepWidth":i32, "Axis 1: speed"=w666:i32, "Axis 1: moving"=w690:bool, "Axis 1: stop detected"=w689:bool, "Axis 1:  sensor error"=w688:bool, "Axis 1: sensor diconnected"=w687:bool, "Axis 2: StepWidth"=→"Axis 2: StepWidth":i32, "Axis 2: Current Position"=→"axis 2:\nCurrent position (°)" →"axis 2:\nCurrent position [µm/°/m°] 2":i32, "Axis 2: speed"=w670:i32, "Axis 2: moving"=w685:bool, "Axis 2: stop detected"=w684:bool, "Axis 2:  sensor error"=w683:bool, "Axis 2: sensor diconnected"=w682:bool, "Axis 2: rot. count"=→"Axis 2: rot. count":i32, "Axis 2: Capacitance"=→"Axis 2: Capacitance [nF]":i32)
            n288 = Bundle("Axis 1: moving"=w690, "Axis 1: stop detected"=w689, "Axis 1:  sensor error"=w688, "Axis 1: sensor diconnected"=w687) -> (→"axis 1:\npositioner status":T12)  [unwired: 1 in]
            n289 = Bundle("Axis 2: moving"=w685, "Axis 2: stop detected"=w684, "Axis 2:  sensor error"=w683, "Axis 2: sensor diconnected"=w682) -> (→"axis 2:\npositioner status":T13)  [unwired: 1 in]
            n290 = To Double Precision Float(number=w666) -> (double precision float=w665:dbl)
            n291 = To Double Precision Float(number=w670) -> (double precision float=w669:dbl)
            n292 = Divide(x=w665, y=1000.0) -> (x/y=w664:dbl)
            n293 = Divide(x=w669, y=1000.0) -> (x/y=w668:dbl)
            n294 = To Long Integer(number=w664) -> (32bit integer=→"Axis 1: speed (°/s)":i32)
            n295 = To Long Integer(number=w668) -> (32bit integer=→"Axis 2: speed (°/s)":i32)
            n296 = call <vilib>:"Add State(s) to Queue__jki_lib_state_machine.vi"("State(s) in (\"\")"=w696) -> ("States Out"=w695:string)  [unwired: 14 in]
          }
          frame "UI: Cursor Set" {
            # "Argument"
            # "Initialize the User Interface, here.\n(this is called automatically, by the Macro: Init)"
            n297 = disable-structure shown="Default" {
              disable-tunnel: w699 -> [w704 w707]
              disable-tunnel: [w704 w706] -> w698
              disable-tunnel: w697 -> [_ w705]
              frame condition #0 {
              }
              frame condition #1 (active) {
                n298 = case shown="\"Busy\"" w705 {
                  tunnel: w707 -> [w709 w711]
                  tunnel: [w708 w710] -> w706
                  frame "Idle", Default {
                    n299 = call <vilib>:"Unset Busy.vi"("error in (no error)"=w709) -> ("error out"=w708:errorcluster)  [unwired: 10 in]
                  }
                  frame "Busy" {
                    n300 = call <vilib>:"Set Busy.vi"("error in (no error)"=w711) -> ("error out"=w710:errorcluster)  [unwired: 9 in, 1 out]
                  }
                }
              }
            }
            n301 = call <vilib>:"Add State(s) to Queue__jki_lib_state_machine.vi"("State(s) in (\"\")"=w703) -> ("States Out"=w702:string)  [unwired: 14 in]
          }
          frame "UI: Front Panel State" {
            # "Argument"
            # "Set Front Panel Open or Closed\n(Usage: \"UI: Front Panel State >> Open|Close\")"
            n302 = Unbundle By Name(w715) -> ("Core.Current VI Reference"=w714:refnum<vi>)
            n303 = disable-structure shown="Default" {
              disable-tunnel: w717 -> [w723 w746]
              disable-tunnel: [w722 w746] -> w716
              disable-tunnel: w714 -> [w721 _]
              disable-tunnel: w713 -> [w720 _]
              frame condition #0 (active) {
                n304 = case shown="\"Close\"" w720 {
                  tunnel: w723 -> [w727 w740]
                  tunnel: [w729 w741] -> w722
                  tunnel: w721 -> [w728 w738]
                  frame "Open", Default {
                    n305 = property class="VI"(reference=w728, error in=w727) -> (reference out=w725:refnum<vi>, error out=w726:errorcluster, "FP.State"=w724:T4)
                    n306 = case shown="\"Closed\"" w724 {
                      tunnel: [w732 w735] -> w729
                      tunnel: w726 -> [w731 w735]
                      tunnel: w725 -> [w730 _]
                      frame "Closed" {
                        n307 = invoke class="VI" method="FP.Open"(reference=w730, error in=w731, "Activate"=TRUE, "State"=T4."Standard") -> (error out=w732:errorcluster)  [unwired: 1 in, 4 out]
                      }
                      frame Default {
                      }
                    }
                  }
                  frame "Close" {
                    n308 = property class="VI"(reference=w738, error in=w740) -> (reference out=w737:refnum<vi>, error out=w739:errorcluster, "FP.State"=w736:T4)
                    n309 = case shown="Default" w736 {
                      tunnel: [w742 w745] -> w741
                      tunnel: w739 -> [w742 w744]
                      tunnel: w737 -> [_ w743]
                      frame "Invalid", "Closed" {
                      }
                      frame Default {
                        n310 = invoke class="VI" method="FP.Close"(reference=w743, error in=w744) -> (error out=w745:errorcluster)  [unwired: 1 in, 2 out]
                      }
                    }
                  }
                }
              }
              frame condition #1 {
              }
            }
            n311 = call <vilib>:"Add State(s) to Queue__jki_lib_state_machine.vi"("State(s) in (\"\")"=w719) -> ("States Out"=w718:string)  [unwired: 14 in]
          }
          frame "---------- Macro ----------" {
            # "Do not put any code in this frame.\n(It is a separator no-op. You can make a copy of this frame to create a new Macro frame)"
            n312 = call <vilib>:"Add State(s) to Queue__jki_lib_state_machine.vi"("State(s) in (\"\")"=w751) -> ("States Out"=w750:string)  [unwired: 14 in]
          }
          frame "Macro: Initialize" {
            w754 = "UI: Initialize\nMacro: Read UI Config\nAction: Open\n//UI: Front Panel State >> Open"  # UI: Initialize Macro: Read UI Config Action: Open //UI: Front Panel State >> Open
            # "Initialization Macro\n(This is called once, when the VI starts)"
            n313 = call <vilib>:"Add State(s) to Queue__jki_lib_state_machine.vi"("State(s) in Front (\"\")"="Data: Initialize\nInitialize Core Data\nEvents: Register", "State(s) in (\"\")"="Process: Sync", "State(s) at Back (\"\")"=w754) -> ("States Out"=w753:string)  [unwired: 12 in]
            n314 = call <vilib>:"Add State(s) to Queue__jki_lib_state_machine.vi"("State(s) in Front (\"\")"=w753, "State(s) in (\"\")"=w760) -> ("States Out"=w759:string)  [unwired: 13 in]
          }
          frame "Macro: Post Error Handling" {
            # "Clear Last Error?"
            n315 = Unbundle By Name(w762) -> ("Core.Last Error.remaining states"=w764:string, "Core.Shutdown?"=w765:bool)
            n316 = Unbundle By Name(w762) -> ("Core.Last Error.error"=w768:errorcluster)
            n317 = case shown="False" FALSE {
              tunnel: w768 -> [w776 _]
              tunnel: [w776 _] -> w767
              frame False {
              }
              frame True {
              }
            }
            n318 = case shown="True" w765 {
              tunnel: w764 -> [w773 w775]
              tunnel: [w773 w774] -> w761
              frame False {
                # "These are the remaining states (at the moment the error occured). States can be altered according to business logic."
                # "NOT SHUTTING DOWN"
              }
              frame True {
                # "Developer can decide to alter the states but should be aware that during the shutdown process, there are certain states that must be run for the SMO to properly shut itself (and this process) down. As such, one can add states to perform additional clean-ups, but should append the remaining state to be executed."
                # "SHUTTING DOWN"
                n319 = call <vilib>:"Add State(s) to Queue__jki_lib_state_machine.vi"("State(s) in (\"\")"=w775) -> ("States Out"=w774:string)  [unwired: 14 in]
              }
            }
            n320 = Bundle By Name(cluster=w762, "Core.Last Error.error"=w767) -> (w763:T10)
            n321 = call <vilib>:"Add State(s) to Queue__jki_lib_state_machine.vi"("State(s) in Front (\"\")"=w761, "State(s) in (\"\")"=w772) -> ("States Out"=w771:string)  [unwired: 13 in]
          }
          frame "Macro: Read UI Config" {
            # "Do not put any code in this frame.\n(It is a separator no-op. You can make a copy of this frame to create a new Macro frame)"
            n322 = call <vilib>:"Add State(s) to Queue__jki_lib_state_machine.vi"("State(s) in Front (\"\")"="Configuration: Initialize\nConfiguration: Read UI Config File\nUI: Update FP Controls" ("State(s) in Front (\"\")"), "State(s) in (\"\")"=w782) -> ("States Out"=w781:string)  [unwired: 13 in]
          }
          frame "Macro: Write UI Config" {
            # "Do not put any code in this frame.\n(It is a separator no-op. You can make a copy of this frame to create a new Macro frame)"
            n323 = call <vilib>:"Add State(s) to Queue__jki_lib_state_machine.vi"("State(s) in Front (\"\")"="Data: Set UI Cluster\nConfiguration: Write UI Config File" ("State(s) in Front (\"\")"), "State(s) in (\"\")"=w788) -> ("States Out"=w787:string)  [unwired: 13 in]
          }
          frame "Macro: Exit" {
            # "Exit Macro\n(This is called once, when the VI exits)"
            n324 = Unbundle By Name(w790) -> ("Core.Close Panel on Exit?"=w800:bool)
            n325 = Select(t="UI: Front Panel State >> Close", s=w800, f="" ("Empty String Constant")) -> (s? t:f=w797:string)
            n326 = call <vilib>:"Add State(s) to Queue__jki_lib_state_machine.vi"("State(s) in Front (\"\")"="Data: Cleanup\nEvents: Unregister\nProcess: Self Terminate", "State(s) in (\"\")"="Process: Sync", "State(s) at Back (\"\")"="Exit") -> ("States Out"=w792:string)  [unwired: 12 in]
            n327 = call <vilib>:"Add State(s) to Queue__jki_lib_state_machine.vi"("State(s) in Front (\"\")"="Action: Close\nMacro: Write UI Config", "State(s) in (\"\")"=w797, "State(s) at Back (\"\")"=w792) -> ("States Out"=w796:string)  [unwired: 12 in]
            n328 = call <vilib>:"Add State(s) to Queue__jki_lib_state_machine.vi"("State(s) in Front (\"\")"=w796, "State(s) in (\"\")"=w803) -> ("States Out"=w802:string)  [unwired: 13 in]
          }
          frame "---------- Process ----------" {
            # "Template Separator\n(You can make a copy of, or modify, this frame)"
            n329 = call <vilib>:"Add State(s) to Queue__jki_lib_state_machine.vi"("State(s) in (\"\")"=w808) -> ("States Out"=w807:string)  [unwired: 14 in]
          }
          frame "Process: Sync" {
            n330 = Unbundle By Name(w816) -> ("Instrument UI"=w812:refnum<class "Inst UI.Attocube-3DR.lvclass">)
            n331 = call <vilib>:"WaitOnProcessSync.vi"("error in (no error)"=w811, "SMO"=w812) -> ("error out"=w810:errorcluster, "Don't run?"=w815:bool)  [unwired: 7 in, 1 out]
            n332 = Select(t="Data: Cleanup\nEvents: Unregister\nExit", s=w815, f="" ("Empty String Constant")) -> (s? t:f=w809:string)
            n333 = call <vilib>:"Add State(s) to Queue__jki_lib_state_machine.vi"("State(s) in Front (\"\")"=w809, "State(s) in (\"\")"=w819) -> ("States Out"=w818:string)  [unwired: 13 in]
          }
          frame "Process: Self Terminate" {
            n334 = Unbundle By Name(w821) -> ("Instrument UI"=w820:refnum<class "Inst UI.Attocube-3DR.lvclass">)
            n335 = call <vilib>:"SelfTerminate.vi"("error in (no error)"=w823, "SMO in"=w820) -> ("error out"=w822:errorcluster)  [unwired: 8 in, 1 out]
            n336 = call <vilib>:"Add State(s) to Queue__jki_lib_state_machine.vi"("State(s) in (\"\")"=w826) -> ("States Out"=w825:string)  [unwired: 14 in]
          }
          frame "---------- Events ----------" {
            # "Template Separator\n(You can make a copy of, or modify, this frame)"
            n337 = call <vilib>:"Add State(s) to Queue__jki_lib_state_machine.vi"("State(s) in (\"\")"=w831) -> ("States Out"=w830:string)  [unwired: 14 in]
          }
          frame "Events: Register" {
            # "Expand to add\nmore events"
            # "Base Class Protected Events"
            n338 = Unbundle By Name(w845) -> ("Instrument UI"=w838:refnum<class "Inst UI.Attocube-3DR.lvclass">, "Instrument"=w837:refnum<class "Inst.Attocube-3DR.lvclass">)
            n339 = call <vilib>:"GetProtectedEvents.vi"("SMO"=w838) -> ("error out"=w841:errorcluster, "SMO Protected Events"=w843:T14)  [unwired: 8 in, 1 out]
            n340 = call <userlib>:"Instrument.GetPublicEvents.vi"("Instrument"=w837) -> ("error out"=w839:errorcluster, "Instrument Public Events"=w840:T15, "Instrument out"=w835:refnum<class "Inst.Attocube-3DR.lvclass">)  [unwired: 8 in]
            n341 = call "Inst.Attocube-3DR.GetPublicEvents.vi"("Inst.Attocube-3DR in"=w835) -> ("error out"=w834:errorcluster, "Inst.Attocube-3DR Public Events"=w836:T16)  [unwired: 8 in, 1 out]
            n342 = register-events(w843, w840, w836) -> (reference out=w844:refnum<event-registration>, error out=w833:errorcluster)  [unwired: 2 in]
            n343 = Merge Errors(w833, w834, w839, w841, w832) -> (w842:errorcluster)
            n344 = call <vilib>:"Add State(s) to Queue__jki_lib_state_machine.vi"("State(s) in (\"\")"=w847) -> ("States Out"=w846:string)  [unwired: 14 in]
          }
          frame "Events: Unregister" {
            n345 = Unregister For Events(event registration refnum=w850, error in=w849) -> (error out=w848:errorcluster)
            n346 = call <vilib>:"Add State(s) to Queue__jki_lib_state_machine.vi"("State(s) in (\"\")"=w853) -> ("States Out"=w852:string)  [unwired: 14 in]
          }
          frame "---------- Configuration ----------" {
            # "Do not put any code in this frame.\n(It is a separator no-op. You can make a copy of this frame to create a new UI frame)"
            n347 = call <vilib>:"Add State(s) to Queue__jki_lib_state_machine.vi"("State(s) in (\"\")"=w858) -> ("States Out"=w857:string)  [unwired: 14 in]
          }
          frame "Configuration: Initialize" {
            # "Do not put any code in this frame.\n(It is a separator no-op. You can make a copy of this frame to create a new UI frame)"
            n348 = Unbundle By Name(w866) -> ("Configuration"=w864:refnum<class "Configuration.lvclass">, "Instrument"=w865:refnum<class "Inst.Attocube-3DR.lvclass">)
            n349 = call <vilib>:"GetName.vi"("error in (no error)"=w868, "SMO"=w865) -> ("error out"=w867:errorcluster, "Name"=w869:string)  [unwired: 6 in, 2 out]
            n350 = call <userlib>:"Default Path.vi"("error in (no error)"=w867, "Folder Name [Application Name]"=w869, "Configuration in"=w864) -> ("error out"=w860:errorcluster, "Configuration out"=w863:refnum<class "Configuration.lvclass">)  [unwired: 7 in]
            n351 = call <userlib>:"Write Section.vi"("error in (no error)"=w860, "Section"="UI", "Configuration in"=w863) -> ("error out"=w859:errorcluster, "Configuration out"=w862:refnum<class "Configuration.lvclass">)  [unwired: 7 in]
            n352 = Bundle By Name(cluster=w866, "Configuration"=w862) -> (w870:T10)
            n353 = call <vilib>:"Add State(s) to Queue__jki_lib_state_machine.vi"("State(s) in (\"\")"=w873) -> ("States Out"=w872:string)  [unwired: 14 in]
          }
          frame "Configuration: Write UI Config File" {
            # "Do not put any code in this frame.\n(It is a separator no-op. You can make a copy of this frame to create a new Data frame)"
            n354 = Unbundle By Name(w878) -> ("Configuration"=w875:refnum<class "Configuration.lvclass">, "UI Cluster"=w877:T8)
            n355 = call <userlib>:"Write Configuration.vi"("error in (no error)"=w874, "Variant"=w877, "Configuration in"=w875) -> ("error out"=w876:errorcluster)  [unwired: 7 in, 1 out]
            n356 = call <vilib>:"Add State(s) to Queue__jki_lib_state_machine.vi"("State(s) in (\"\")"=w881) -> ("States Out"=w880:string)  [unwired: 14 in]
          }
          frame "Configuration: Read UI Config File" {
            # "Do not put any code in this frame.\n(It is a separator no-op. You can make a copy of this frame to create a new UI frame)"
            n357 = Unbundle By Name(w884) -> ("UI Cluster"=w887:T8, "Configuration"=w890:refnum<class "Configuration.lvclass">)
            n358 = call <userlib>:"Read Configuration.vi"("INI Fomatted Cluster Type"=w887, "error in (no error)"=w886, "Configuration in"=w890) -> ("error out"=w889:errorcluster, "Configuration"=w888:variant)  [unwired: 6 in, 1 out]
            n359 = Variant To Data(error in=w889, type=w887, Variant=w888) -> (data=w883:T8, error out=w885:errorcluster)
            n360 = Bundle By Name(cluster=w884, "UI Cluster"=w883) -> (w882:T10)
            n361 = call <vilib>:"Add State(s) to Queue__jki_lib_state_machine.vi"("State(s) in (\"\")"=w893) -> ("States Out"=w892:string)  [unwired: 14 in]
          }
          frame "---------- Action ----------" {
            n362 = Unbundle By Name(w895) -> ("Instrument"=w896:refnum<class "Inst.Attocube-3DR.lvclass">)
            n363 = Bundle By Name(cluster=w895, "Instrument"=w896) -> (w894:T10)
            n364 = call <vilib>:"Add State(s) to Queue__jki_lib_state_machine.vi"("State(s) in (\"\")"=w900) -> ("States Out"=w899:string)  [unwired: 14 in]
          }
          frame "Action: Notify UI Closed" {
            # "Notify that the UI has been closed"
            n365 = Unbundle By Name(w901) -> ("Instrument UI"=w904:refnum<class "Inst UI.Attocube-3DR.lvclass">)
            n366 = call <vilib>:"Hide.vi"("error in (no error)"=w903, "SMO.UI"=w904) -> ("error out"=w902:errorcluster)  [unwired: 8 in, 1 out]
            n367 = call <vilib>:"Add State(s) to Queue__jki_lib_state_machine.vi"("State(s) in (\"\")"=w907) -> ("States Out"=w906:string)  [unwired: 14 in]
          }
          frame "Action: getAll" {
            n368 = Unbundle By Name(w911) -> ("getAll"=w909:T7, "Instrument"=w914:refnum<class "Inst.Attocube-3DR.lvclass">)
            n369 = call "GET ALL.vim"("type"=w909, "error in (no error)"=w912, "Instrument in"=w914) -> ("error out"=w916:errorcluster, "getAll"=w908:T7, "Instrument out"=w910:refnum<class "Inst.Attocube-3DR.lvclass">)  [unwired: 6 in]
            n370 = Bundle By Name(cluster=w911, "Instrument"=w910, "getAll"=w908) -> (w913:T10)
            n371 = call <vilib>:"Add State(s) to Queue__jki_lib_state_machine.vi"("State(s) in Front (\"\")"="" ("State(s) in Front (\"\")"), "State(s) in (\"\")"=w919) -> ("States Out"=w918:string)  [unwired: 13 in]
          }
          frame "Action: Open" {
            n372 = Unbundle By Name(w926) -> ("Instrument"=w924:refnum<class "Inst.Attocube-3DR.lvclass">)
            n373 = call <userlib>:"Write Client Type.vi"("error in (no error)"=w921, "Client Type"=Client_Type--Enum."Local", "Instrument in"=w924) -> ("error out"=w922:errorcluster, "Instrument out"=w923:refnum<class "Inst.Attocube-3DR.lvclass">)  [unwired: 7 in]
            n374 = call-dynamic "Open.vi"("error in (no error)"=w922, "Inst.Attocube-3DR in"=w923) -> ("error out"=w929:errorcluster, "Inst.Attocube-3DR out"=w925:refnum<class "Inst.Attocube-3DR.lvclass">)  [unwired: 8 in]
            n375 = Bundle By Name(cluster=w926, "Instrument"=w925) -> (w927:T10)
            n376 = call <vilib>:"Add State(s) to Queue__jki_lib_state_machine.vi"("State(s) in Front (\"\")"="" ("State(s) in Front (\"\")"), "State(s) in (\"\")"=w932) -> ("States Out"=w931:string)  [unwired: 13 in]
          }
          frame "Action: Close" {
            n377 = Unbundle By Name(w934) -> ("Instrument"=w937:refnum<class "Inst.Attocube-3DR.lvclass">)
            n378 = call-dynamic "Close.vi"("error in (no error)"=w935, "Inst.Attocube-3DR in"=w937) -> ("error out"=w939:errorcluster, "Inst.Attocube-3DR out"=w933:refnum<class "Inst.Attocube-3DR.lvclass">)  [unwired: 8 in]
            n379 = Bundle By Name(cluster=w934, "Instrument"=w933) -> (w936:T10)
            n380 = call <vilib>:"Add State(s) to Queue__jki_lib_state_machine.vi"("State(s) in Front (\"\")"="" ("State(s) in Front (\"\")"), "State(s) in (\"\")"=w942) -> ("States Out"=w941:string)  [unwired: 13 in]
          }
          frame "Action: Send Message to Instrument" {
            # "Send a message (command, data, etc) to the Instrument:process.vi"
            n381 = Unbundle By Name(w949) -> ("Instrument"=w948:refnum<class "Inst.Attocube-3DR.lvclass">, "Message.Command"=w944:string, "Message.Data"=w943:variant)
            n382 = call <userlib>:"Instrument.MessageToProcess.vi"("error in (no error)"=w946, "Data"=w943, "Command"=w944, "Instrument"=w948) -> ("error out"=w945:errorcluster, "Instrument out"=w947:refnum<class "Inst.Attocube-3DR.lvclass">)  [unwired: 6 in]
            n383 = Bundle By Name(cluster=w949, "Instrument"=w947) -> (w950:T10)
            n384 = call <vilib>:"Add State(s) to Queue__jki_lib_state_machine.vi"("State(s) in Front (\"\")"="" ("State(s) in Front (\"\")"), "State(s) in (\"\")"=w954) -> ("States Out"=w953:string)  [unwired: 13 in]
          }
          frame "Action: Send Message to Child" {
            # "Send a message (command, data, etc) to the Instrument.Child:process.vi"
            n385 = Unbundle By Name(w961) -> ("Instrument"=w960:refnum<class "Inst.Attocube-3DR.lvclass">, "Message.Data"=w955:variant, "Message.Command"=w956:string)
            n386 = call "Inst.Attocube-3DR.MessageToProcess.vi"("error in (no error)"=w958, "Data"=w955, "Command"=w956, "Inst.Attocube-3DR in"=w960) -> ("error out"=w957:errorcluster, "Inst.Attocube-3DR out"=w959:refnum<class "Inst.Attocube-3DR.lvclass">)  [unwired: 6 in]
            n387 = Bundle By Name(cluster=w961, "Instrument"=w959) -> (w962:T10)
            n388 = call <vilib>:"Add State(s) to Queue__jki_lib_state_machine.vi"("State(s) in Front (\"\")"="" ("State(s) in Front (\"\")"), "State(s) in (\"\")"=w966) -> ("States Out"=w965:string)  [unwired: 13 in]
          }
        }
      }
    }
    frame Error {
    }
  }
  n389 = call-parent "Process.vi"("error in"=w5, "Instrument UI in"=w4) -> ("error out"=w2:errorcluster, "Instrument UI out"=→"Inst UI.Attocube-3DR out":refnum<class "Inst UI.Attocube-3DR.lvclass">)  [unwired: 8 in]
  n390 = Merge Errors(w2, w1) -> (→"error out":errorcluster)
